vi "CPP-Multiplot.vi"(0 "PlotArray":cluster{dbl[], dbl[]}[](array[cluster]), 1 "Job Directory":path) -> (2 "Saved Automatically?":bool, 3 "gnuplotScript":string, 4 "Plot data file":path)   [LabVIEW 2015]
uses:
  gnuplotScriptComponents/plotstyle.ctl
  gnuplotScriptComponents/graphPeripherals.ctl
  gnuplotScriptComponents/minAndMax.ctl
  gnuplotScriptComponents/AutoManualNumber.ctl
  gnuplotScriptComponents/ticsAndGrids.ctl
  gnuplotScriptComponents/tics.ctl
  gnuplotScriptComponents/grids.ctl
  gnuplotScriptComponents/legendProperties.ctl
  gnuplotScriptComponents/legendAppearance.ctl
  gnuplotScriptComponents/alignment.ctl
  gnuplotScriptComponents/at.ctl
  gnuplotScriptComponents/margins.ctl
  gnuplotScriptComponents/source.ctl
  gnuplotScriptComponents/Master_Legend.ctl
  gnuplotScriptComponents/MasterPeripherals.ctl
  gnuplotScriptComponents/axisName.ctl
  Results_plotter_Global.vi
panel:
  in  "ThetaLabelCMD":string="rmax = GPVAL_R_MAX\nrmin = GPVAL_R_MIN\nThetaLabelPosn = rmax + (rmax - rmin) * 0.1\ndo for [jip = 0:17]{\nthetaer = jip*20\ntexter = sprintf(\"%.0f\",thetaer)\nset_label(x,text) = sprintf(\"set label '%s%s' at (-ThetaLabelPosn*cos(90+%f)), (ThetaLabelPosn*sin(90+%f)) center\", texter,\"$^{o}$\", thetaer, thetaer)\neval set_label(thetaer,texter)\n}\nset multiplot previous\n\nreplot\n\nunset label\n"
  out "Multi_Plot":bool
  in  "OpenLogfile?":bool
  in  "Show Script Editor?":bool
  in  "Tab Control":T1(tab)=enum."Appearance"
  in  "Each Graph contains:":T2=enum."Series"
  in  "Rows from:":T2=enum."Until done"
  in  "Columns from:":T2=enum."Selector 1"
  in  "Margins":T3={"Top"=2.0, "Bottom"=2.0, "Left"=2.0, "Right"=2.0}
  in  "Height (in)":dbl=7.0 min=0.5 step=0.5 format="%.1f"
  in  "Width (in)":dbl=10.0 min=0.5 step=0.5 format="%.1f"
  in  "nRows":u8=3 min=1
  in  "nCols":u8=3 min=1
  in  "ScaleAdjust":dbl=0.9 min=0.1 max=2.0 step=0.1
  in  "PlotTitlesNeed $$?":bool=TRUE
  in  "Show Channels with range of Values?":bool
  in  "ManualPlotTitles":string[](array[string])
  out "AutoPlotTitles":string[](array[string])
  in  "Individual Plot Titles":bool=TRUE
  in  "Page Title Pre Block":string
  in  "Page Title Post Block":string
  in  "Values to include in Page Title":i32[](listbox)
  in  "Plot Title Offset (characters)":cluster{"horizontal":dbl, "vertical":dbl}
  out "Final Title":string
  in  "PlotNamesNeed $$?":bool=TRUE
  in  "Plot Legends Manual":string[](array[string])
  in  "Plotstyles":T4[](array[typedef])=[{"Style"="linespoints", "Color"=16711680, "PointType"=1, "PointSize"=1.0, "LineWidth"=1.0, "LineType"=1}, {"Style"="linespoints", "Color"=16860, "PointType"=2, "PointSize"=1.0, "LineWidth"=1.0, "LineType"=1}, {"Style"="linespoints", "Color"=51228, "PointType"=3, "PointSize"=1.0, "LineWidth"=1.0, "LineType"=1}, {"Style"="linespoints", "Color"=0, "PointType"=4, "PointSize"=1.0, "LineWidth"=1.0, "LineType"=1}, {"Style"="linespoints", "Color"=9567230, "PointType"=5, "PointSize"=1.0, "LineWidth"=1.0, "LineType"=1}, {"Style"="linespoints", "Color"=12369084, "PointType"=6, "PointSize"=1.0, "LineWidth"=1.0, "LineType"=1}, {"Style"="linespoints", "Color"=15667967, "PointType"=7, "PointSize"=1.0, "LineWidth"=1.0, "LineType"=1}, {"Style"="linespoints", "Color"=15400704, "PointType"=8, "PointSize"=1.0, "LineWidth"=1.0, "LineType"=1}, {"Style"="linespoints", "Color"=128, "PointType"=9, "PointSize"=1.0, "LineWidth"=1.0, "LineType"=1}, {"Style"="linespoints", "Color"=8404992, "PointType"=10, "PointSize"=1.0, "LineWidth"=1.0, "LineType"=1}, {"Style"="linespoints", "Color"=6737151, "PointType"=11, "PointSize"=1.0, "LineWidth"=1.0, "LineType"=1}, {"Style"="linespoints", "Color"=8388672, "PointType"=12, "PointSize"=1.0, "LineWidth"=1.0, "LineType"=1}, {"Style"="linespoints", "Color"=16740303, "PointType"=13, "PointSize"=1.0, "LineWidth"=1.0, "LineType"=1}, {"Style"="linespoints", "Color"=16764006, "PointType"=14, "PointSize"=1.0, "LineWidth"=1.0, "LineType"=1}, {"Style"="linespoints", "Color"=8421376, "PointType"=15, "PointSize"=1.0, "LineWidth"=1.0, "LineType"=1}, {"Style"="linespoints", "Color"=65408, "PointType"=16, "PointSize"=1.0, "LineWidth"=1.0, "LineType"=1}] caption="Style                      Colour    PointType       PointSize         Linewidth        Linestyle" {"LineType" min=1 max=6 step=1; "LineWidth" min=1 max=6 step=1; "PointSize" min=0 step=0.1}
  out "Plot Legends Auto":string[](array[string])
  out "No of Series supplied":i32
  out "No of Graph Slots Available":i32
  in  "Plot Legends":bool=TRUE
  in  "X axis label":enum32{"Autolabel", "Manual Label"}(tab)
  out "X or theta label":string
  in  "X or theta label Manual":string
  in  "LegendProperties":T5={"Appearance"={"layout"="", "text-sample order"="", "key order"="", "surroundingBox"="", "MaxRows"=0, "MaxCols"=0, "WidthAdjust"=0.0}, "Alignment"={"Horizontal"="", "Vertical"=""}, "Location"="auto", "\"At\" location"={"XcoordSys"="", "YcoordSys"="", "Xvalue"=0.0, "Yvalue"=0.0}}
  in  "Y/R tics And Grids":T9={"tics"={"ticMin"=0.0, "ticStep"=5.0, "ticMax"=0.0, "minorDivsPerMajor"=2, "ticSpacing"=enum."Approx n Tics (rounded)", "ticPosition"=enum."Inside, no mirror"}, "Grids"={"Gridlines"=enum."No grids", "Zeroaxis"=enum."No zero axis"}, "Mapping"=enum."Lin"}
  in  "X/Theta tics And Grids":T9={"tics"={"ticMin"=0.0, "ticStep"=5.0, "ticMax"=0.0, "minorDivsPerMajor"=2, "ticSpacing"=enum."Approx n Tics (rounded)", "ticPosition"=enum."Inside, no mirror"}, "Grids"={"Gridlines"=enum."Major grid", "Zeroaxis"=enum."No zero axis"}, "Mapping"=enum."Lin"}
  in  "PlotType":enum32{"XY", "Polar", "Time"}(tab)
  in  "yAxisBounds":T12={"Min"={"Auto"=TRUE, "Value"=0.0}, "Max"={"Auto"=TRUE, "Value"=0.0}}
  in  "Additional XYgnuplot":string
  in  "xAxisBounds":T12={"Min"={"Auto"=TRUE, "Value"=0.0}, "Max"={"Auto"=TRUE, "Value"=0.0}}
  in  "Set bounds using XY Plot \non Results file plotter":bool
  in  "Angle Units":bool=TRUE
  in  "AngleMode":string(combo)="Compass"
  in  "wrapGapsUpTo:":dbl=30.0 step=0.1
  in  "Additional Polar gnuplot":string
  in  "rAxisBounds":T12={"Min"={"Auto"=FALSE, "Value"=0.0}, "Max"={"Auto"=FALSE, "Value"=1.5}}
  out "Time format?":bool
  in  "Time/Date Format":string(combo)="%I:%M %p\\n%d-%b-%y"
  in  "Select Time Zone":u32(ring)=142 items=["Abbreviation (Time Zone Name)", "A (Alpha Time Zone)", "ACDT (Australian Central Daylight Time  CDT – Central Daylight Time CDST – Central Daylight Savings Time)", "ACST (Australian Central Standard Time  CST – Central Standard Time)", "ACT (Acre Time)", "ACT (Australian Central Time)", "ACWST (Australian Central Western Standard Time)", "ADT (Arabia Daylight Time  AST – Arabia Summer Time)", "ADT (Atlantic Daylight Time  ADST – Atlantic Daylight Saving Time AST – Atlantic Summer Time  HAA – Heure Avancée de l'Atlantique (French))", "AEDT (Australian Eastern Daylight Time  EDT – Eastern Daylight Time EDST – Eastern Daylight Saving Time)", "AEST (Australian Eastern Standard Time  EST – Eastern Standard Time AET – Australian Eastern Time)", "AET (Australian Eastern Time)", "AFT (Afghanistan Time)", "AKDT (Alaska Daylight Time  ADST – Alaska Daylight Saving Time)", "AKST (Alaska Standard Time  AT – Alaska Time)", "ALMT (Alma-Ata Time)", "AMST (Amazon Summer Time)", "AMST (Armenia Summer Time  AMDT – Armenia Daylight Time)", "AMT (Amazon Time)", "AMT (Armenia Time)", "ANAST (Anadyr Summer Time)", "ANAT (Anadyr Time)", "AQTT (Aqtobe Time)", "ART (Argentina Time)", "AST (Arabia Standard Time  AST – Arabic Standard Time AST – Al Manamah Standard Time)", "AST (Atlantic Standard Time  AT – Atlantic Time  AST – Tiempo Estándar del Atlántico (Spanish) HNA – Heure Normale de l'Atlantique (French))", "AT (Atlantic Time)", "AWDT (Australian Western Daylight Time  WDT – Western Daylight Time WST – Western Summer Time)", "AWST (Australian Western Standard Time  WST – Western Standard Time WAT – Western Australia Time)", "AZOST (Azores Summer Time  AZODT – Azores Daylight Time)", "AZOT (Azores Time  AZOST – Azores Standard Time)", "AZST (Azerbaijan Summer Time)", "AZT (Azerbaijan Time)", "AoE (Anywhere on Earth)", "B (Bravo Time Zone)", "BNT (Brunei Darussalam Time  BDT – Brunei Time)", "BOT (Bolivia Time)", "BRST (Brasília Summer Time  BST – Brazil Summer Time BST – Brazilian Summer Time)", "BRT (Brasília Time  BT – Brazil Time BT – Brazilian Time)", "BST (Bangladesh Standard Time)", "BST (Bougainville Standard Time)", "BST (British Summer Time  BDT – British Daylight Time BDST – British Daylight Saving Time)", "BTT (Bhutan Time)", "C (Charlie Time Zone)", "CAST (Casey Time)", "CAT (Central Africa Time)", "CCT (Cocos Islands Time)", "CDT (Central Daylight Time  CDST – Central Daylight Saving Time NACDT – North American Central Daylight Time  HAC – Heure Avancée du Centre (French))", "CDT (Cuba Daylight Time)", "CEST (Central European Summer Time  CEDT – Central European Daylight Time ECST – European Central Summer Time  MESZ – Mitteleuropäische Sommerzeit (German))", "CET (Central European Time  ECT – European Central Time CET – Central Europe Time  MEZ – Mitteleuropäische Zeit (German))", "CHADT (Chatham Island Daylight Time  CDT – Chatham Daylight Time)", "CHAST (Chatham Island Standard Time)", "CHOST (Choibalsan Summer Time  CHODT – Choibalsan Daylight Time CHODST – Choibalsan Daylight Saving Time)", "CHOST (Choibalsan Summer Time)", "CHOT (Choibalsan Time)", "CHUT (Chuuk Time)", "CIDST (Cayman Islands Daylight Saving Time)", "CIST (Cayman Islands Standard Time  CIT – Cayman Islands Time)", "CKT (Cook Island Time)", "CLST (Chile Summer Time  CLDT – Chile Daylight Time)", "CLT (Chile Standard Time  CT – Chile Time CLST – Chile Standard Time)", "COT (Colombia Time)", "CST (Central Standard Time  CT – Central Time NACST – North American Central Standard Time  CST – Tiempo Central Estándar (Spanish) HNC – Heure Normale du Centre (French))", "CST (China Standard Time)", "CST (Cuba Standard Time)", "CT (Central Time)", "CVT (Cape Verde Time)", "CXT (Christmas Island Time)", "ChST (Chamorro Standard Time  GST – Guam Standard Time)", "D (Delta Time Zone)", "DAVT (Davis Time)", "DDUT (Dumont-d'Urville Time)", "E (Echo Time Zone)", "EASST (Easter Island Summer Time  EADT – Easter Island Daylight Time)", "EAST (Easter Island Standard Time)", "EAT (Eastern Africa Time  EAT – East Africa Time)", "ECT (Ecuador Time)", "EDT (Eastern Daylight Time  EDST – Eastern Daylight Savings Time NAEDT – North American Eastern Daylight Time  HAE – Heure Avancée de l'Est (French) EDT – Tiempo de verano del Este (Spanish))", "EEST (Eastern European Summer Time  EEDT – Eastern European Daylight Time  OESZ – Osteuropäische Sommerzeit (German))", "EET (Eastern European Time  OEZ – Osteuropäische Zeit (German))", "EGST (Eastern Greenland Summer Time  EGST – East Greenland Summer Time)", "EGT (East Greenland Time  EGT – Eastern Greenland Time)", "EST (Eastern Standard Time  ET – Eastern Time  NAEST – North American Eastern Standard Time  ET – Tiempo del Este (Spanish) HNE – Heure Normale de l'Est (French))", "ET (Eastern Time)", "F (Foxtrot Time Zone)", "FET (Further-Eastern European Time)", "FJST (Fiji Summer Time  FJDT – Fiji Daylight Time)", "FJT (Fiji Time)", "FKST (Falkland Islands Summer Time  FKDT – Falkland Island Daylight Time)", "FKT (Falkland Island Time  FKST – Falkland Island Standard Time)", "FNT (Fernando de Noronha Time)", "G (Golf Time Zone)", "GALT (Galapagos Time)", "GAMT (Gambier Time  GAMT – Gambier Islands Time)", "GET (Georgia Standard Time)", "GFT (French Guiana Time)", "GILT (Gilbert Island Time)", "GMT (Greenwich Mean Time  \"– Coordinated Universal Time GT – Greenwich Time)", "GST (Gulf Standard Time)", "GST (South Georgia Time)", "GYT (Guyana Time)", "H (Hotel Time Zone)", "HADT (Hawaii-Aleutian Daylight Time  HDT – Hawaii Daylight Time)", "HAST (Hawaii-Aleutian Standard Time  HST – Hawaii Standard Time)", "HKT (Hong Kong Time)", "HOVST (Hovd Summer Time  HOVDT – Hovd Daylight Time HOVDST – Hovd Daylight Saving Time)", "HOVST (Hovd Summer Time)", "HOVT (Hovd Time)", "I (India Time Zone)", "ICT (Indochina Time)", "IDT (Israel Daylight Time)", "IOT (Indian Chagos Time)", "IRDT (Iran Daylight Time  IRST – Iran Summer Time IDT – Iran Daylight Time)", "IRKST (Irkutsk Summer Time)", "IRKT (Irkutsk Time)", "IRST (Iran Standard Time  IT – Iran Time)", "IST (India Standard Time  IT – India Time IST – Indian Standard Time)", "IST (Irish Standard Time  IST – Irish Summer Time)", "IST (Israel Standard Time)", "JST (Japan Standard Time)", "K (Kilo Time Zone)", "KGT (Kyrgyzstan Time)", "KOST (Kosrae Time)", "KRAST (Krasnoyarsk Summer Time)", "KRAT (Krasnoyarsk Time)", "KST (Korea Standard Time  KST – Korean Standard Time KT – Korea Time)", "KUYT (Kuybyshev Time  SAMST – Samara Summer Time)", "L (Lima Time Zone)", "LHDT (Lord Howe Daylight Time)", "LHST (Lord Howe Standard Time)", "LINT (Line Islands Time)", "M (Mike Time Zone)", "MAGST (Magadan Summer Time  MAGST – Magadan Island Summer Time)", "MAGT (Magadan Time  MAGT – Magadan Island Time)", "MART (Marquesas Time)", "MAWT (Mawson Time)", "MDT (Mountain Daylight Time  MDST – Mountain Daylight Saving Time NAMDT – North American Mountain Daylight Time  HAR – Heure Avancée des Rocheuses (French))", "MHT (Marshall Islands Time)", "MMT (Myanmar Time)", "MSD (Moscow Daylight Time  Moscow Summer Time)", "MSK (Moscow Standard Time  MCK – Moscow Time)", "MST (Mountain Standard Time  MT – Mountain Time NAMST – North American Mountain Standard Time  HNR – Heure Normale des Rocheuses (French))", "MT (Mountain Time)", "MUT (Mauritius Time)", "MVT (Maldives Time)", "MYT (Malaysia Time  MST – Malaysian Standard Time)", "N (November Time Zone)", "NCT (New Caledonia Time)", "NDT (Newfoundland Daylight Time  HAT – Heure Avancée de Terre-Neuve (French))", "NFT (Norfolk Time  NFT – Norfolk Island Time)", "NOVST (Novosibirsk Summer Time  OMSST – Omsk Summer Time)", "NOVT (Novosibirsk Time  OMST – Omsk Standard Time)", "NPT (Nepal Time)", "NRT (Nauru Time)", "NST (Newfoundland Standard Time  HNT – Heure Normale de Terre-Neuve (French))", "NUT (Niue Time)", "NZDT (New Zealand Daylight Time)", "NZST (New Zealand Standard Time)", "O (Oscar Time Zone)", "OMSST (Omsk Summer Time  NOVST – Novosibirsk Summer Time)", "OMST (Omsk Standard Time  OMST – Omsk Time NOVT – Novosibirsk Time)", "ORAT (Oral Time)", "P (Papa Time Zone)", "PDT (Pacific Daylight Time  PDST – Pacific Daylight Saving Time NAPDT – North American Pacific Daylight Time  HAP – Heure Avancée du Pacifique (French))", "PET (Peru Time)", "PETST (Kamchatka Summer Time)", "PETT (Kamchatka Time  PETT – Petropavlovsk-Kamchatski Time)", "PGT (Papua New Guinea Time)", "PHOT (Phoenix Island Time)", "PHT (Philippine Time  PST – Philippine Standard Time)", "PKT (Pakistan Standard Time  PKT – Pakistan Time)", "PMDT (Pierre & Miquelon Daylight Time)", "PMST (Pierre & Miquelon Standard Time)", "PONT (Pohnpei Standard Time)", "PST (Pacific Standard Time  PT – Pacific Time NAPST – North American Pacific Standard Time  PT – Tiempo del Pacífico (Spanish) HNP – Heure Normale du Pacifique (French))", "PST (Pitcairn Standard Time)", "PT (Pacific Time)", "PWT (Palau Time)", "PYST (Paraguay Summer Time)", "PYT (Paraguay Time)", "PYT (Pyongyang Time  PYST – Pyongyang Standard Time)", "PYT (Pyongyang Time)", "Q (Quebec Time Zone)", "QYZT (Qyzylorda Time)", "R (Romeo Time Zone)", "RET (Reunion Time)", "ROTT (Rothera Time)", "S (Sierra Time Zone)", "SAKT (Sakhalin Time)", "SAMT (Samara Time  SAMT – Samara Standard Time)", "SAST (South Africa Standard Time  SAST – South African Standard Time)", "SBT (Solomon Islands Time  SBT – Solomon Island Time)", "SCT (Seychelles Time)", "SGT (Singapore Time  SST – Singapore Standard Time)", "SRET (Srednekolymsk Time)", "SRT (Suriname Time)", "SST (Samoa Standard Time)", "SYOT (Syowa Time)", "T (Tango Time Zone)", "TAHT (Tahiti Time)", "TFT (French Southern and Antarctic Time  KIT – Kerguelen (Islands) Time)", "TJT (Tajikistan Time)", "TKT (Tokelau Time)", "TLT (East Timor Time)", "TMT (Turkmenistan Time)", "TOT (Tonga Time)", "TVT (Tuvalu Time)", "U (Uniform Time Zone)", "ULAST (Ulaanbaatar Summer Time  ULAST – Ulan Bator Summer Time)", "ULAST (Ulaanbaatar Summer Time)", "ULAT (Ulaanbaatar Time  ULAT – Ulan Bator Time)", "ULAT (Ulaanbaatar Time)", "UTC (Coordinated Universal Time)", "UYST (Uruguay Summer Time)", "UYT (Uruguay Time)", "UZT (Uzbekistan Time)", "V (Victor Time Zone)", "VET (Venezuelan Standard Time  HLV – Hora Legal de Venezuela (Spanish))", "VLAST (Vladivostok Summer Time)", "VLAT (Vladivostok Time)", "VOST (Vostok Time)", "VUT (Vanuatu Time  EFATE – Efate Time)", "W (Whiskey Time Zone)", "WAKT (Wake Time)", "WARST (Western Argentine Summer Time)", "WAST (West Africa Summer Time)", "WAT (West Africa Time)", "WEST (Western European Summer Time  WEDT – Western European Daylight Time  WESZ – Westeuropäische Sommerzeit (German))", "WET (Western European Time  GMT – Greenwich Mean Time  WEZ – Westeuropäische Zeit (German))", "WFT (Wallis and Futuna Time)", "WGST (Western Greenland Summer Time  WGST – West Greenland Summer Time)", "WGT (West Greenland Time  WGT – Western Greenland Time)", "WIB (Western Indonesian Time  WIB – Waktu Indonesia Barat)", "WIT (Eastern Indonesian Time  WIT – Waktu Indonesia Timur)", "WITA (Central Indonesian Time  WITA – Waktu Indonesia Tengah)", "WST (West Samoa Time  ST – Samoa Time)", "WST (Western Sahara Summer Time)", "WT (Western Sahara Standard Time  WT – Western Sahara Time)", "X (X-ray Time Zone)", "Y (Yankee Time Zone)", "YAKST (Yakutsk Summer Time)", "YAKT (Yakutsk Time)", "YAPT (Yap Time)", "YEKST (Yekaterinburg Summer Time)", "YEKT (Yekaterinburg Time)", "Z (Zulu Time Zone)"]
  out "Time Format String":string="%I:%M %p\\n%d-%b-%y"
  out "Formatted date/time string":string="05:00 PM\\n21-Jan-16"
  out "TZ Shift (hrs)":string="UTC-7.00"
  in  "Y axis label":enum32{"Autolabel", "Manual Label"}(tab)
  out "Y or R label":string
  in  "Y or R label Manual 2":string
  in  "PeripheralsMasterControl":T14=enum."Edges Only"
  in  "Legend Options":T15=enum."Single Legend Below table"
  in  "GraphPeripherals":T16[][](array[typedef])
  out "PlotCommand":string
  in  "Filename Max length":i32=255
  out "File Path Control":path
  out "AuditTrail":string[](array[string])
  out "Desired Legends":string[][](array[string])
  out "original name had conflict":bool
  out "crossplatform problem":bool
  # "Rows/ Columns/ Series from: controls not wired- just a thought for explicit control of what goes where...?"
  # "Overall Page Title"
  # "There are as many graphs as there are titles (from Selector 2)...."
  # "Plot Styles"
  # "Each graph contains plots from Selector 1..."
  # "X/theta"
  # "Y/r"
  # "Shows the numbered line colours and point styles available- well it would, if it didn't disappear every time I update from the repository..!"
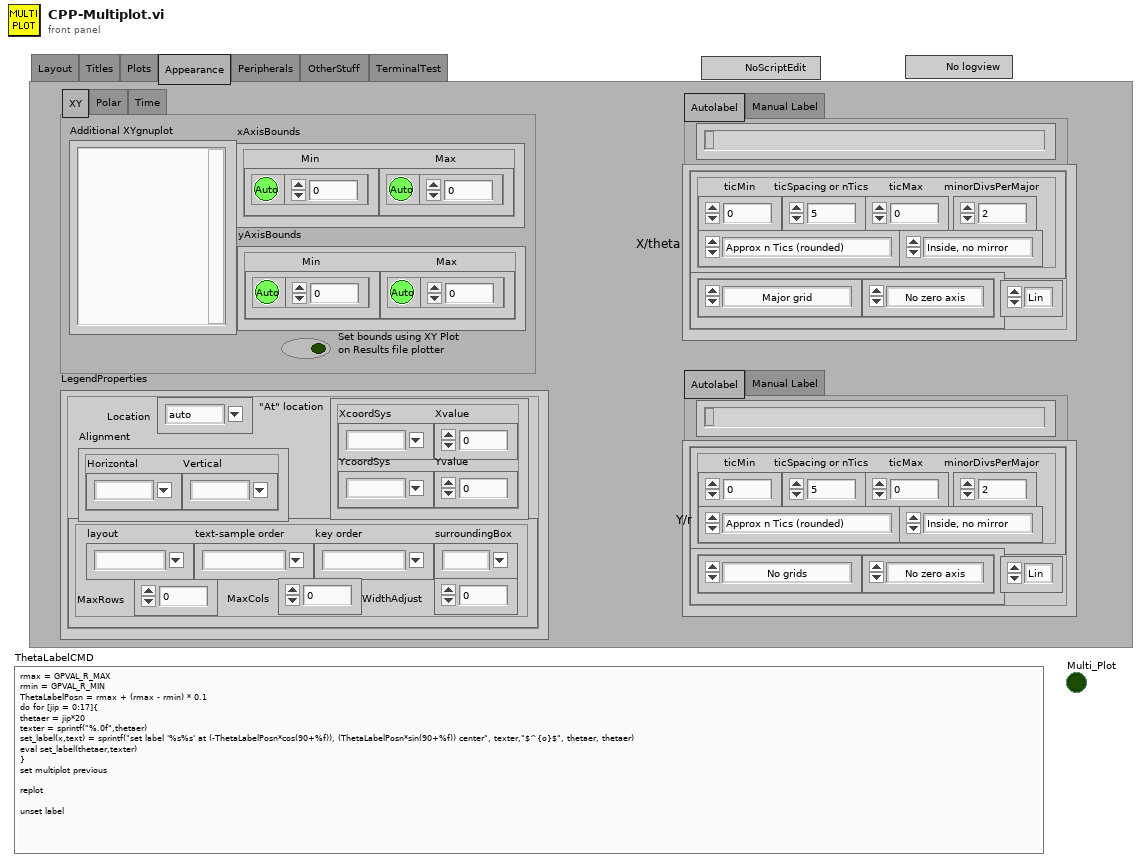
[diagram p1: front panel]
types:
  T1 = enum32{"Layout", "Titles", "Plots", "Appearance", "Peripherals", "OtherStuff ", "TerminalTest"}
  T2 = typedef "source.ctl" = enum16{"Specified:", "Selector 1", "Selector 2", "Until done", "Series"}
  T3 = typedef "margins.ctl" = cluster{"Top":dbl, "Bottom":dbl, "Left":dbl, "Right":dbl}
  T4 = typedef "plotstyle.ctl" = cluster{"Style":string, "Color":u32, "PointType":i32, "PointSize":sgl, "LineWidth":sgl, "LineType":u8}
  T5 = typedef "legendProperties.ctl" = cluster{"Appearance":T6, "Alignment":T7, "Location":string, "\"At\" location":T8}
  T6 = typedef "legendAppearance.ctl" = cluster{"layout":string, "text-sample order":string, "key order":string, "surroundingBox":string, "MaxRows":u32, "MaxCols":u32, "WidthAdjust":dbl}
  T7 = typedef "alignment.ctl" = cluster{"Horizontal":string, "Vertical":string}
  T8 = typedef "at.ctl" = cluster{"XcoordSys":string, "YcoordSys":string, "Xvalue":dbl, "Yvalue":dbl}
  T9 = typedef "ticsAndGrids.ctl" = cluster{"tics":T10, "Grids":T11, "Mapping":enum8{"Lin", "Log"}}
  T10 = typedef "tics.ctl" = cluster{"ticMin":dbl, "ticStep":dbl, "ticMax":dbl, "minorDivsPerMajor":i32, "ticSpacing":enum16{"Auto Tics", "Fixed spacing", "Fixed Minimum and Spacing", "Start, Spacing and Maximum", "Approx n Tics (rounded)"}, "ticPosition":enum16{"Inside, no mirror", "Inside, mirrored", "Outside, no mirror", "Outside, mirrored", "Invisible"}}
  T11 = typedef "grids.ctl" = cluster{"Gridlines":enum16{"No grids", "Major grid", "Minor grid", "Major and Minor"}, "Zeroaxis":enum16{"No zero axis", "Show zero axis"}}
  T12 = typedef "minAndMax.ctl" = cluster{"Min":T13, "Max":T13}
  T13 = typedef "AutoManualNumber.ctl" = cluster{"Auto":bool, "Value":dbl}
  T14 = typedef "MasterPeripherals.ctl" = enum16{"Use Table", "Titles On", "Edges Only", "All Off"}
  T15 = typedef "Master_Legend.ctl" = enum16{"No Legend", "Single Legend Below table", "Legend as per array"}
  T16 = typedef "graphPeripherals.ctl" = cluster{"title":bool, "key":bool, "Xtic":bool, "Ytic":bool, "Xlab":bool, "Ylab":bool}
  T17 = typedef "axisName.ctl" = string
  T18 = typedef "LVDateTimeRec.ctl" = cluster{"fractional second":dbl, "second":i32, "minute":i32, "hour":i32, "day of month":i32, "month":i32, "year":i32, "day of week":i32, "day of year":i32, "DST":i32}
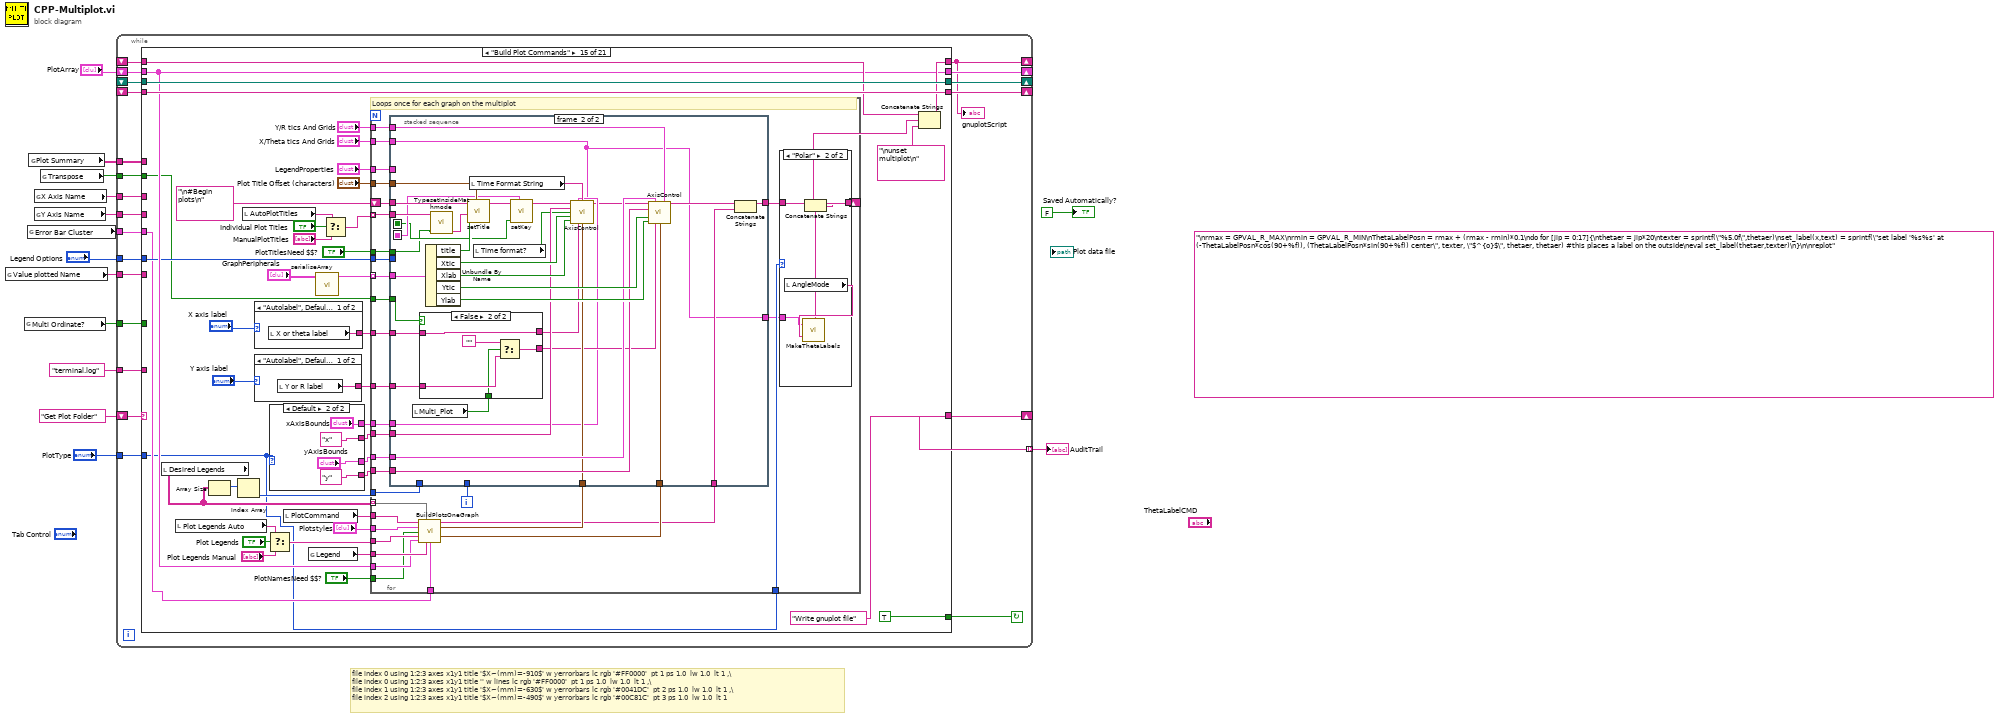
[diagram p0: block diagram]
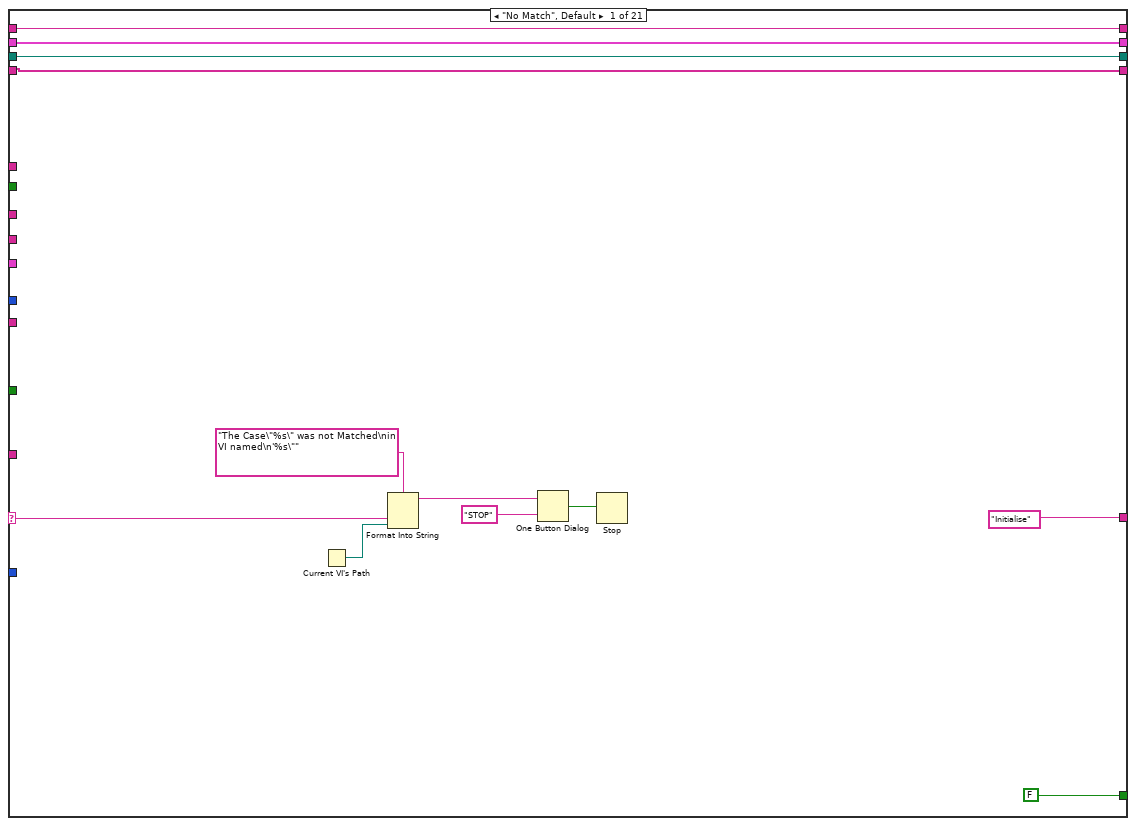
[diagram p2: hidden frame]
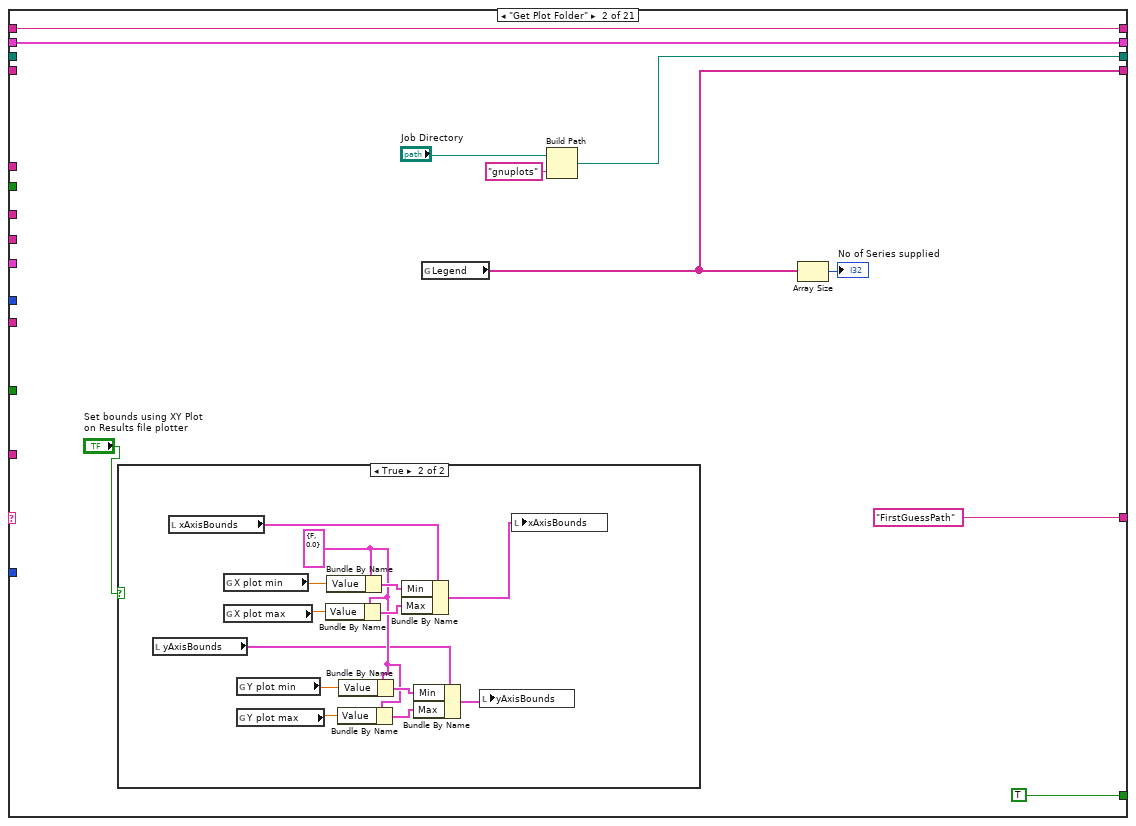
[diagram p3: hidden frame]
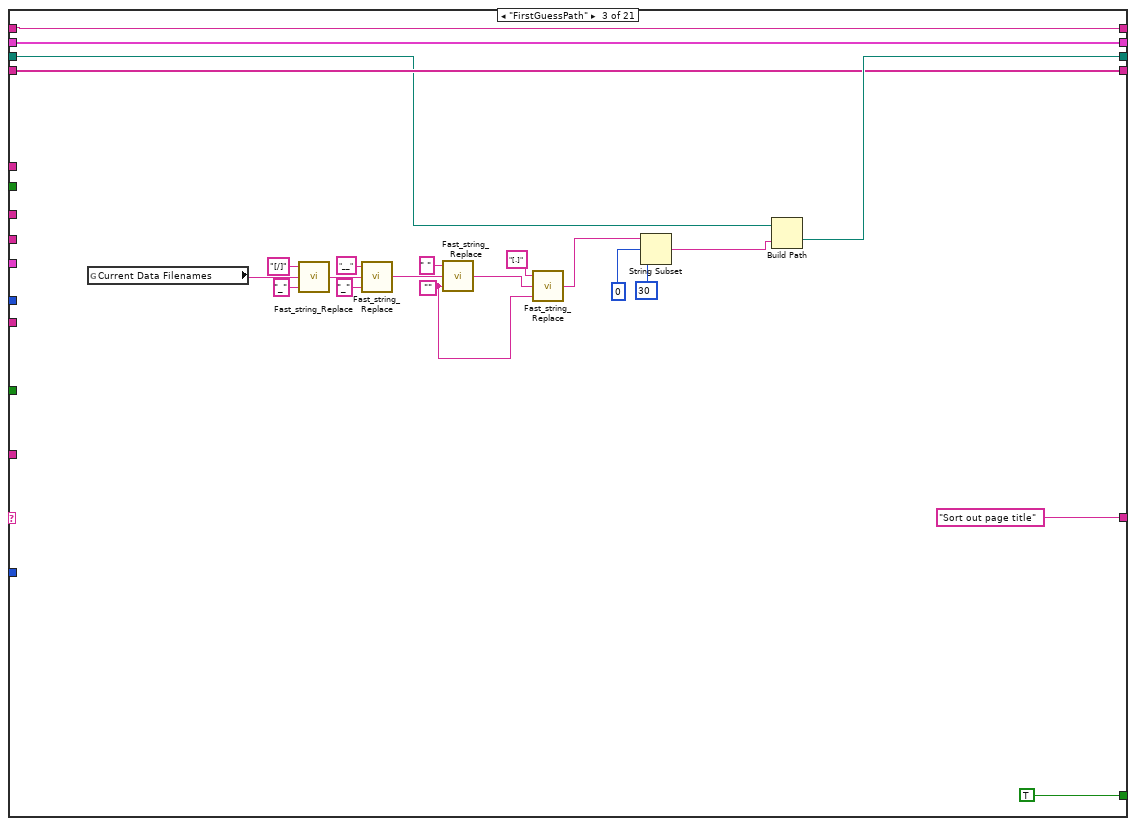
[diagram p5: hidden frame]
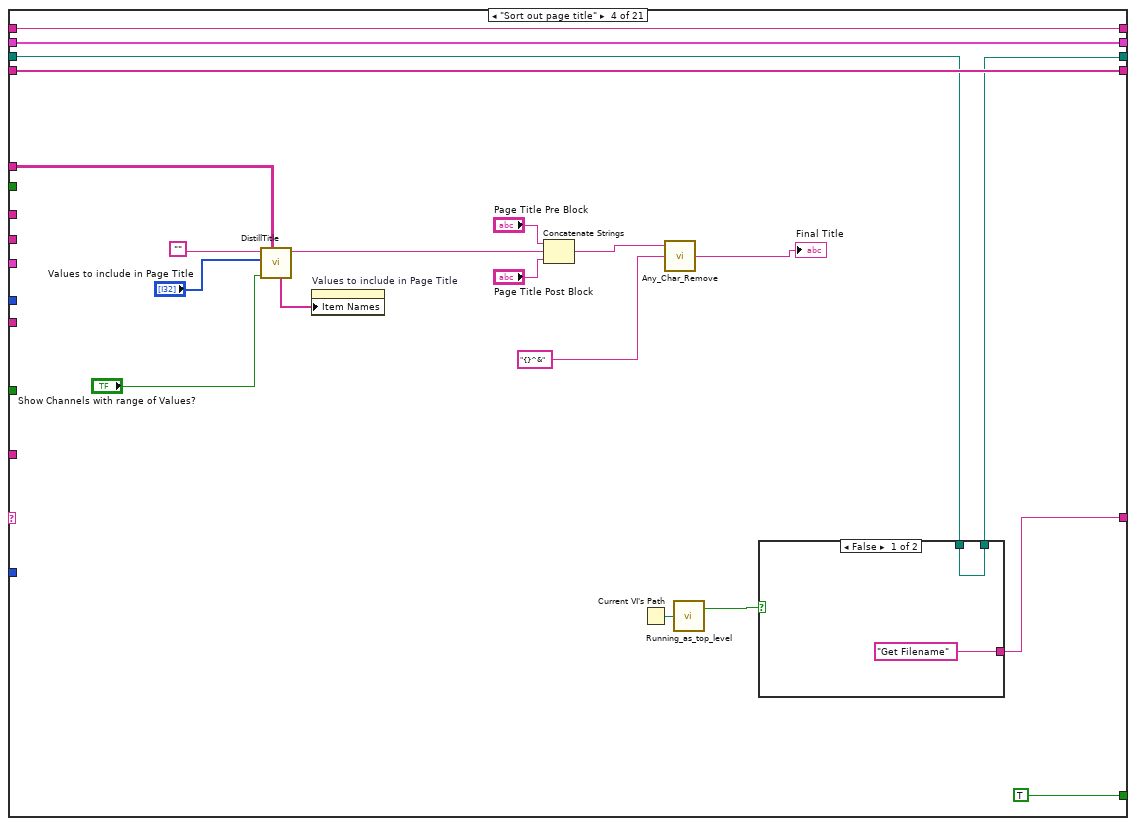
[diagram p6: hidden frame]
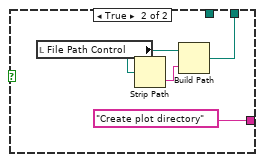
[diagram p7: hidden frame]
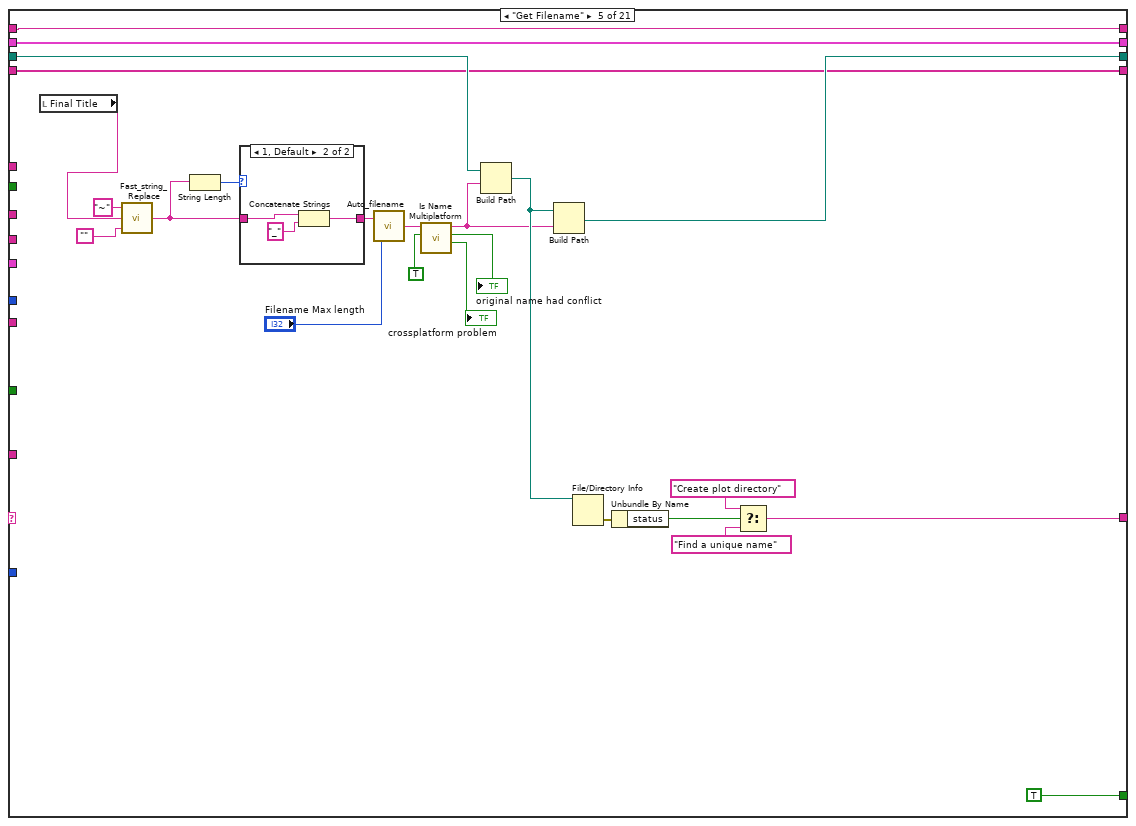
[diagram p8: hidden frame]
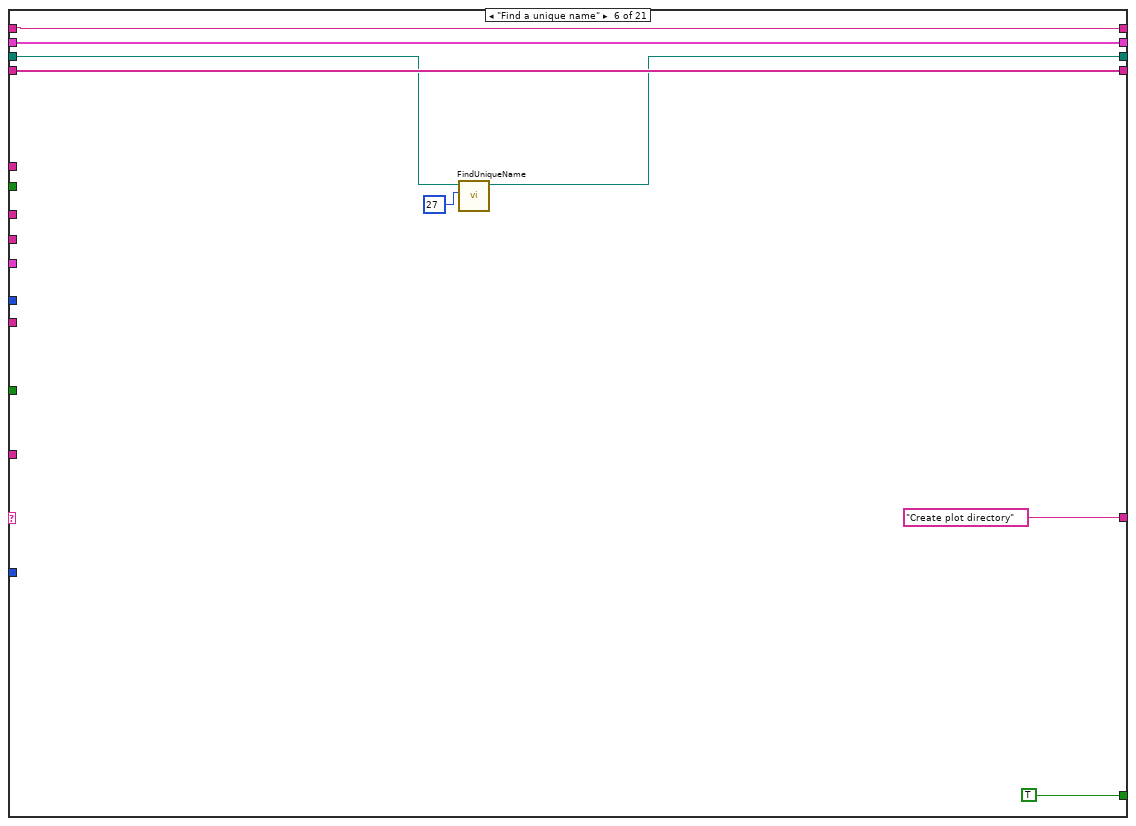
[diagram p10: hidden frame]
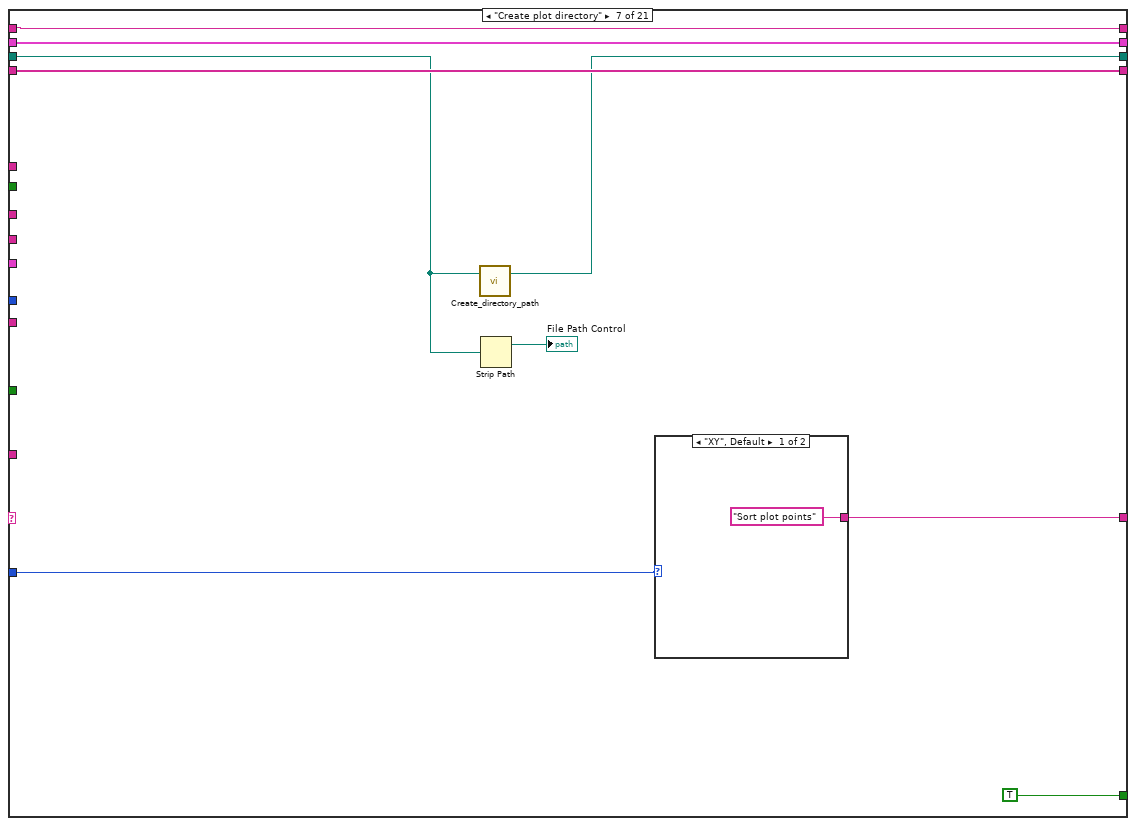
[diagram p11: hidden frame]
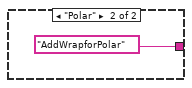
[diagram p12: hidden frame]
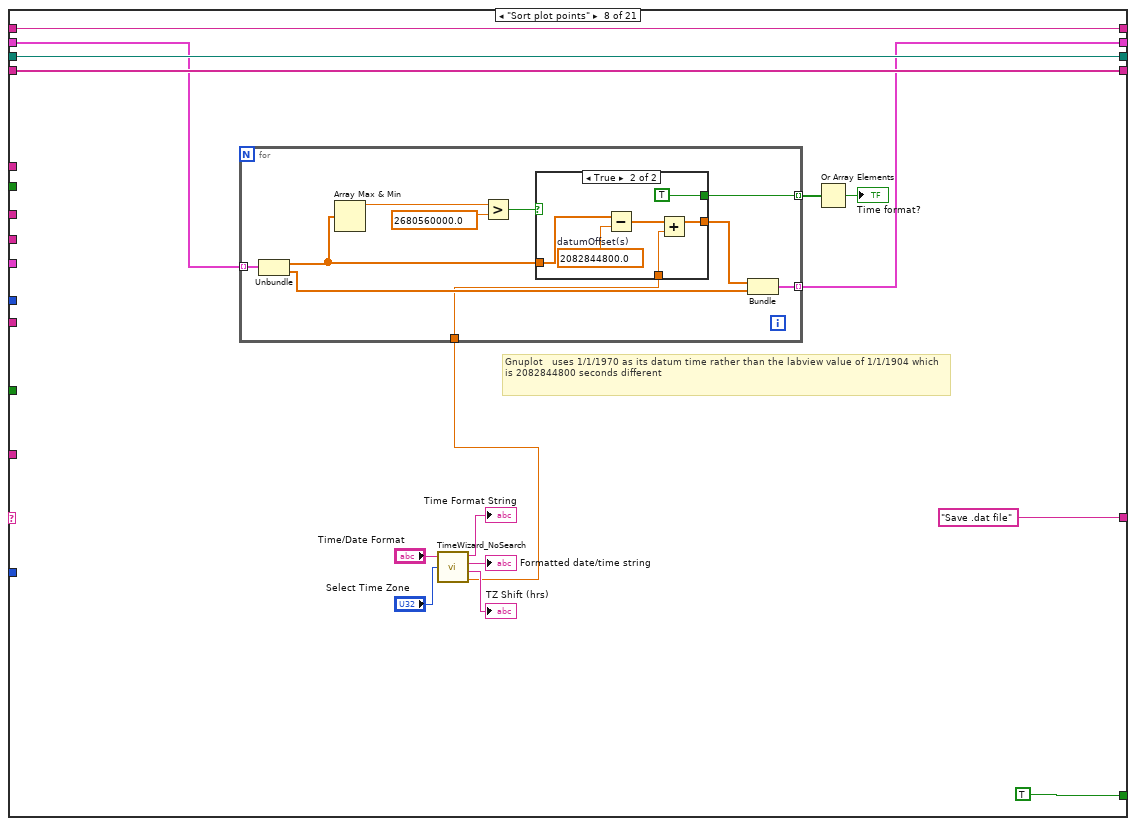
[diagram p13: hidden frame]
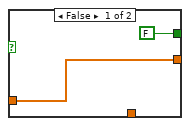
[diagram p14: hidden frame]
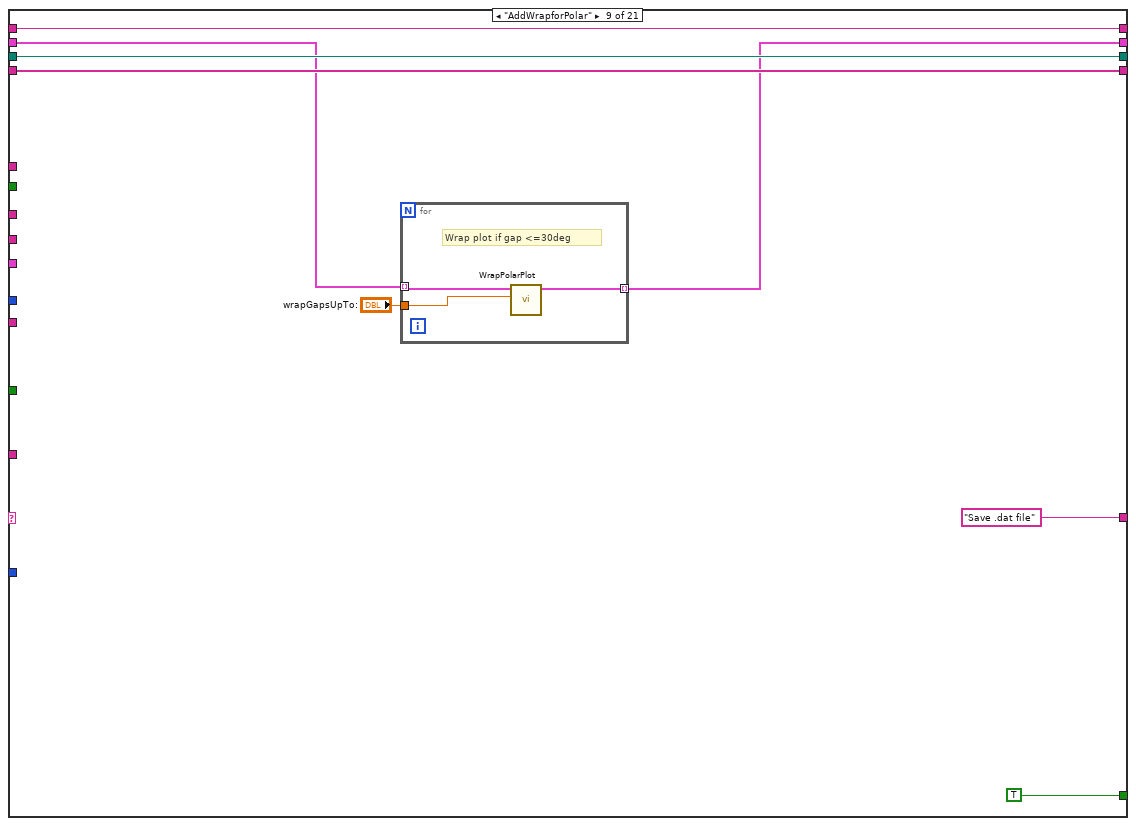
[diagram p15: hidden frame]
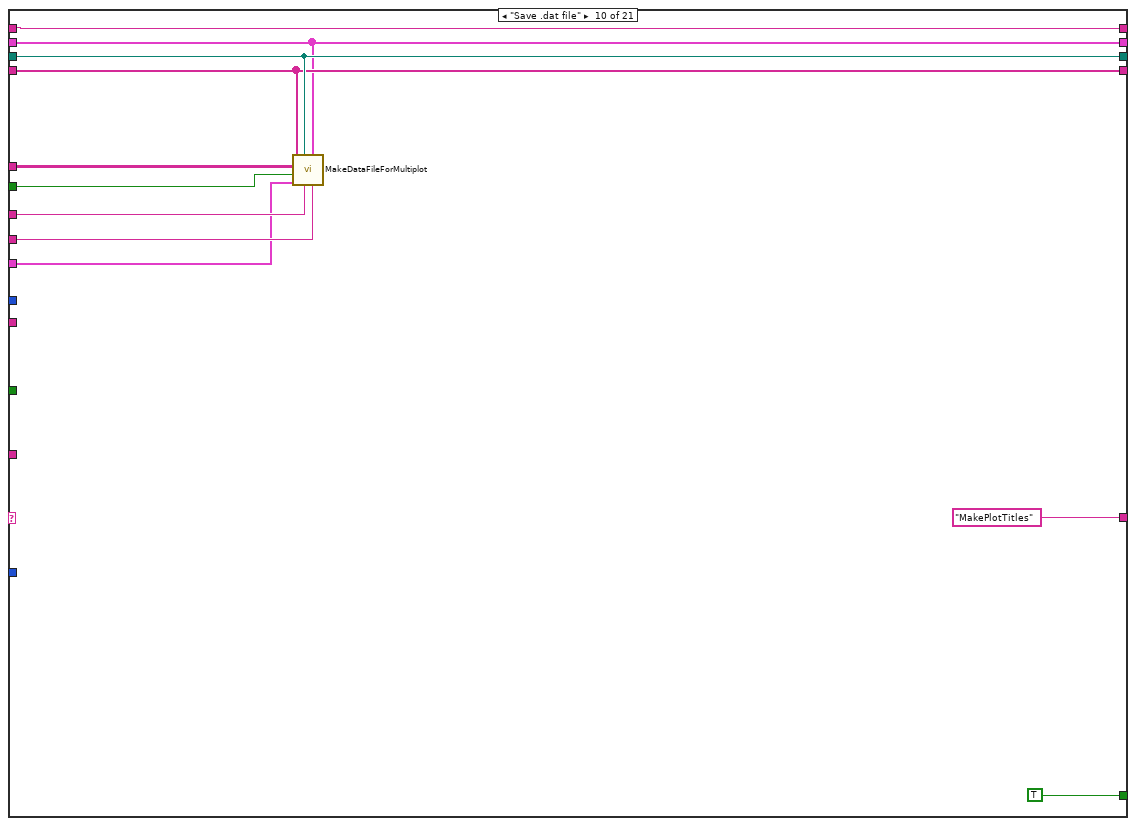
[diagram p16: hidden frame]
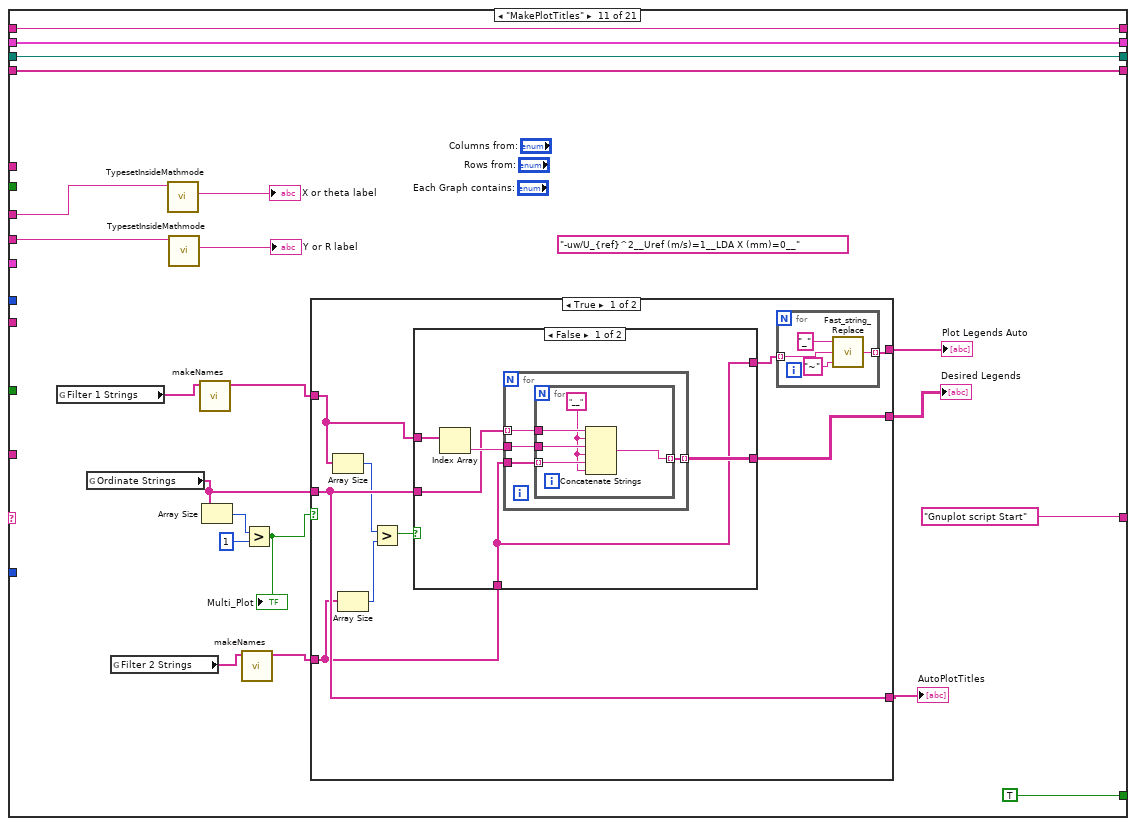
[diagram p17: hidden frame]
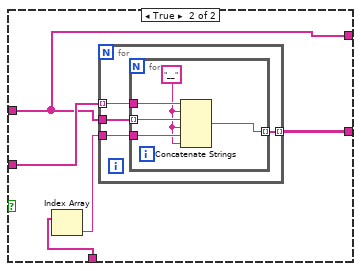
[diagram p18: hidden frame]
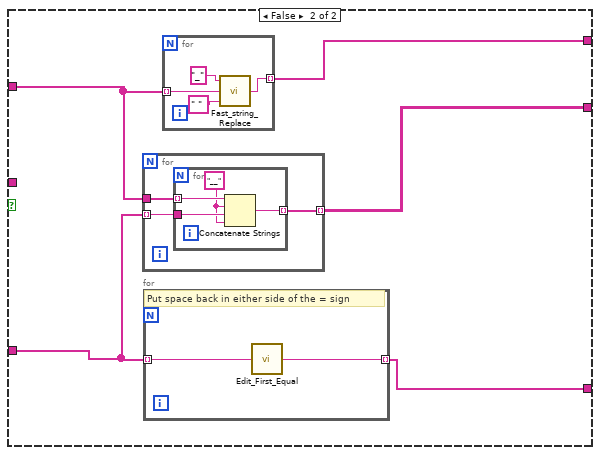
[diagram p19: hidden frame]
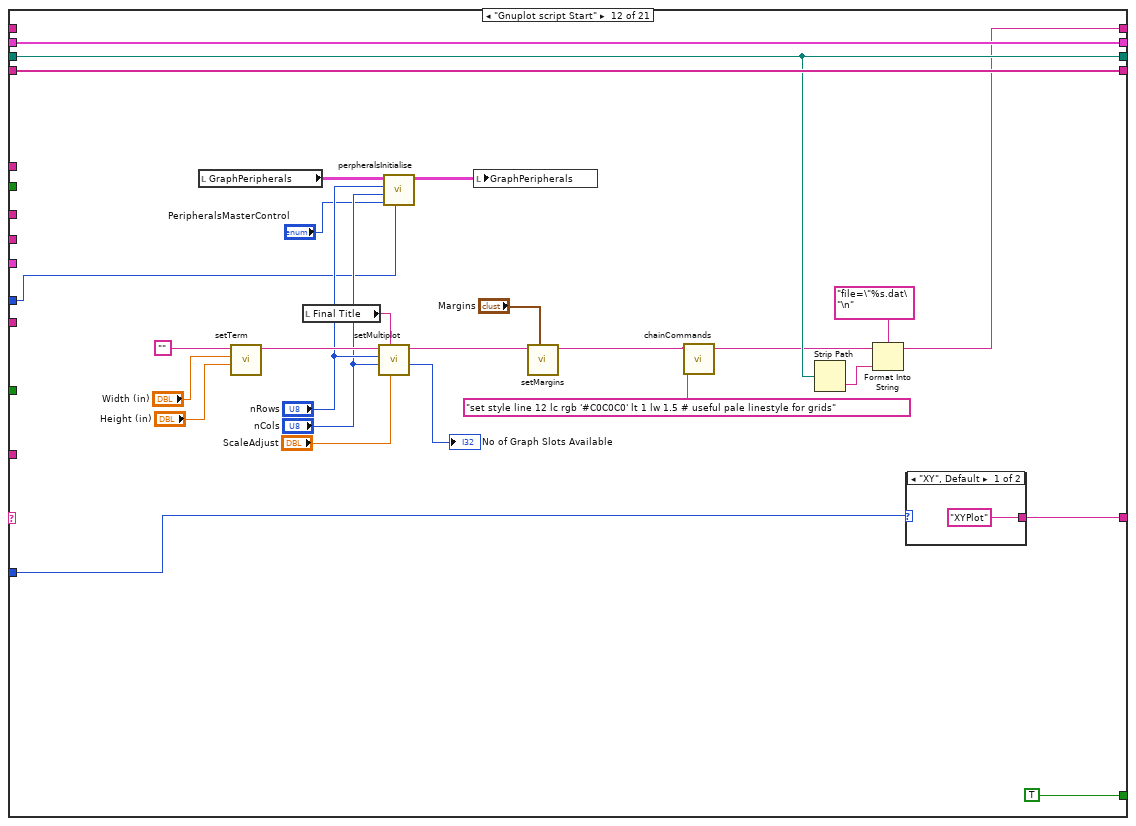
[diagram p20: hidden frame]
diagram:
  (unwired) "\nrmax = GPVAL_R_MAX\nrmin = GPVAL_R_MIN\nThetaLabelPosn = rmax + (rmax - rmin)*0.1\ndo for [jip = 0:17]{\nthetaer = jip*20\ntexter = sprintf(\"%5.0f\",thetaer)\nset_label(x,text) = sprintf(\"set label '%s%s' at (-ThetaLabelPosn*cos(90+%f)), (ThetaLabelPosn*sin(90+%f)) center\", texter, \"$^{o}$\", thetaer, thetaer) #this places a label on the outside\neval set_label(thetaer,texter)\n}\n\nreplot" ("string")
  # "file index 0 using 1:2:3 axes x1y1 title '$X~(mm)=-910$' w yerrorbars lc rgb '#FF0000'  pt 1 ps 1.0  lw 1.0  lt 1 ,\\\nfile index 0 using 1:2:3 axes x1y1 title '' w lines lc rgb '#FF0000'  pt 1 ps 1.0  lw 1.0  lt 1 ,\\\nfile index 1 using 1:2:3 axes x1y1 title '$X~(mm)=-630$' w yerrorbars lc rgb '#0041DC'  pt 2 ps 1.0  lw 1.0  lt 1 ,\\\nfile index 2 using 1:2:3 axes x1y1 title '$X~(mm)=-490$' w yerrorbars lc rgb '#00C81C'  pt 3 ps 1.0  lw 1.0  lt 1"
  n1 = global read "Results_plotter_Global.vi" "Value plotted Name"() -> (w10:string)
  n2 = global read "Results_plotter_Global.vi" "Multi Ordinate?"() -> (w6:bool)
  n3 = global read "Results_plotter_Global.vi" "Error Bar Cluster"() -> (w1:cluster{string[]}[])
  n4 = global read "Results_plotter_Global.vi" "Plot Summary"() -> (w13:string[][])
  n5 = global read "Results_plotter_Global.vi" "X Axis Name"() -> (w12:string)
  n6 = global read "Results_plotter_Global.vi" "Y Axis Name"() -> (w11:string)
  n7 = global read "Results_plotter_Global.vi" "Transpose"() -> (w7:bool)
  n8 = while {
    shift-left: "Get Plot Folder" -> [w34]
    shift-right: [w18] -> _
    tunnel: w13 -> [w33]
    shift-right: [w32] -> _
    shift-left: _ -> [w31]
    tunnel: w12 -> [w30]
    tunnel: w11 -> [w29]
    tunnel: w10 -> [w28]
    shift-right: [w26] -> _
    shift-left: "PlotArray" -> [w27]
    shift-right: [w19] -> _
    shift-left: _ -> [w25]
    shift-right: [w24] -> _
    shift-left: _ -> [w23]
    tunnel: "terminal.log" -> [w22]
    tunnel: w7 -> [w21]
    tunnel: w6 -> [w20]
    tunnel: [w18] -> w5 mode=indexing
    tunnel: "PlotType" -> [w17]
    tunnel: "Legend Options" -> [w16]
    tunnel: w1 -> [w15]
    stop <- w35 continue-if-true
    n9 = case shown="\"Build Plot Commands\"" w34 {
      selector: w34 -> [w36 _ _ _ _ _ _ _ _ _ _ _ _ _ _ _ _ _ _ _ _]
      tunnel: [FALSE TRUE TRUE ("Top Level") TRUE ("Top Level") TRUE ("Top Level") TRUE ("Top Level") TRUE TRUE TRUE ("Top Level") TRUE ("Top Level") TRUE ("Top Level") TRUE ("Top Level") TRUE ("Top Level") TRUE ("Top Level") TRUE ("Top Level") TRUE ("Top Level") TRUE ("Top Level") TRUE ("Top Level") FALSE ("Top Level") TRUE ("Top Level") FALSE ("Top Level")] -> w35
      tunnel: ["Initialise" "FirstGuessPath" "Sort out page title" w104 w140 "Create plot directory" w155 "Save .dat file" "Save .dat file" "MakePlotTitles" "Gnuplot script Start" w324 "Build Plot Commands" "Build Plot Commands" "Write gnuplot file" ("t") "Execute shell script" ("t") "Has pdf been generated?" ("t") w602 "End" "End" ("t") "End" ("t")] -> w18
      tunnel: w33 -> [_ _ _ w99 _ _ _ _ _ w218 _ _ _ _ _ _ _ _ _ _ _]
      tunnel: [w40 w55 w92 w106 w141 w147 w160 w180 w205 w219 w241 w315 w340 w366 w420 w560 w568 w597 w615 w625 w636] -> w32
      tunnel: w31 -> [w40 _ w88 w105 w137 w148 w159 w180 w205 w219 w241 w315 w340 w366 w420 w560 w568 w597 w615 w625 w636]
      tunnel: w30 -> [_ _ _ _ _ _ _ _ _ w217 w235 _ _ _ _ _ _ _ _ _ _]
      tunnel: w29 -> [_ _ _ _ _ _ _ _ _ w216 w234 _ _ _ _ _ _ _ _ _ _]
      tunnel: w28 -> [_ _ _ _ _ _ _ _ _ _ _ _ _ _ _ _ _ _ _ _ _]
      tunnel: w27 -> [w39 w51 w91 w112 w139 w151 w163 w175 w201 w213 w240 w327 w339 w367 w388 w566 w573 w608 w620 w630 w635]
      tunnel: [w39 w51 w91 w112 w139 w151 w163 w174 w200 w213 w240 w327 w339 w367 w388 w566 w573 w608 w620 w630 w635] -> w26
      tunnel: w25 -> [w38 w54 w90 w110 w138 w150 w162 w179 w206 w220 w239 _ w333 w361 w412 w556 w571 w606 w618 w628 w634]
      tunnel: [w38 w54 w90 w110 w138 w150 w162 w179 w206 w220 w239 w301 w335 w362 w418 w556 w571 w606 w618 w628 w634] -> w19
      tunnel: [w37 w50 w89 w111 w136 w149 w161 w178 w204 w215 w238 w326 w338 w365 w419 w561 w572 w607 w619 w629 w633] -> w24
      tunnel: w23 -> [w37 _ w89 w111 w136 w149 w161 w178 w204 w215 w238 w326 w338 w365 w419 w561 w572 w607 w619 w629 w633]
      tunnel: w22 -> [_ _ _ _ _ _ _ _ _ _ _ _ _ _ _ _ w567 _ _ w623 _]
      tunnel: w21 -> [_ _ _ _ _ _ _ _ _ w214 _ _ _ _ w384 _ _ _ _ _ _]
      tunnel: w20 -> [_ _ _ _ _ _ _ _ _ _ _ _ _ _ _ _ _ _ _ _ _]
      tunnel: w17 -> [_ _ _ _ _ _ w156 _ _ _ _ w302 _ _ w377 _ _ _ _ _ _]
      tunnel: w16 -> [_ _ _ _ _ _ _ _ _ _ _ w304 _ _ w387 _ _ _ _ _ _]
      tunnel: w15 -> [_ _ _ _ _ _ _ _ _ w210 _ _ _ _ w385 _ _ _ _ _ _]
      frame "No Match", Default {
        n10 = Current VI's Path() -> (path=w42:path)
        n11 = Format Into String(format string="The Case\"%s\" was not Matched\nin VI named\n'%s\"" ("Format String"), w36, w42) -> (resulting string=w45:string)  [unwired: 2 in, 1 out]
        n12 = One Button Dialog(message=w45, button name ("OK")="STOP") -> (true=w43:bool)
        n13 = Stop(stop? (T)=w43) -> ()
      }
      frame "Get Plot Folder" {
        n14 = case shown="True" "Set bounds using XY Plot \non Results file plotter" {
          frame False {
          }
          frame True {
            w60 = T13 {"Auto"=FALSE, "Value"=0.0} ("Min")
            n15 = local read "yAxisBounds"() -> (w59:T12)
            n16 = local read "xAxisBounds"() -> (w70:T12)
            n17 = global read "Results_plotter_Global.vi" "X plot min"() -> (w65:dbl)
            n18 = global read "Results_plotter_Global.vi" "X plot max"() -> (w66:dbl)
            n19 = global read "Results_plotter_Global.vi" "Y plot min"() -> (w64:dbl)
            n20 = global read "Results_plotter_Global.vi" "Y plot max"() -> (w63:dbl)
            n21 = Bundle By Name(cluster=w60, "Value"=w66) -> (w68:T13)
            n22 = Bundle By Name(cluster=w60, "Value"=w65) -> (w69:T13)
            n23 = Bundle By Name(cluster=w60, "Value"=w63) -> (w62:T13)
            n24 = Bundle By Name(cluster=w60, "Value"=w64) -> (w61:T13)
            n25 = Bundle By Name(cluster=w70, "Min"=w69, "Max"=w68) -> (w67:T12)
            n26 = Bundle By Name(cluster=w59, "Min"=w61, "Max"=w62) -> (w58:T12)
            n27 = local write "yAxisBounds"(w58) -> ()
            n28 = local write "xAxisBounds"(w67) -> ()
          }
        }
        n29 = global read "Results_plotter_Global.vi" "Legend"() -> (w50:string[])
        n30 = Build Path(base path="Job Directory", name or relative path="gnuplots") -> (appended path=w55:path)
        n31 = Array Size(array=w50) -> (size(s)=→"No of Series supplied":i32)
      }
      frame "FirstGuessPath" {
        w74 = ""
        n32 = global read "Results_plotter_Global.vi" "Current Data Filenames"() -> (w78:string)
        n33 = call "Fast_string_Replace.vi"("Replace match with:"="_", "Input String"=w78, "regular expression"="[/]") -> ("Output String"=w81:string)  [unwired: 2 out]
        n34 = call "Fast_string_Replace.vi"("Replace match with:"="_", "Input String"=w81, "regular expression"="__") -> ("Output String"=w79:string)  [unwired: 2 out]
        n35 = call "Fast_string_Replace.vi"("Replace match with:"=w74, "Input String"=w79, "regular expression"=" ") -> ("Output String"=w73:string)  [unwired: 2 out]
        n36 = call "Fast_string_Replace.vi"("Replace match with:"=w74, "Input String"=w73, "regular expression"="[.]") -> ("Output String"=w72:string)  [unwired: 2 out]
        n37 = String Subset(string=w72, offset (0)=0, length (rest)=30 ("length (rest)")) -> (substring=w71:string)
        n38 = Build Path(base path=w88, name or relative path=w71) -> (appended path=w92:path)
      }
      frame "Sort out page title" {
        n39 = call "DistillTitle.vi"("Plot Summary in"=w99, "Show Channels with range of Values?"="Show Channels with range of Values?", "Indices to include in Page Title"="Values to include in Page Title", "String in"="") -> ("String out"=w103:string, "AvailableVariables"=w97:string[])  [unwired: 6 in]
        n40 = property on="Values to include in Page Title" class="LstBox (strict)"("Item Names"=w97) -> ()  [unwired: 2 in, 2 out]
        n41 = Concatenate Strings("Page Title Pre Block", w103, "Page Title Post Block") -> (w96:string)
        n42 = Current VI's Path() -> (path=w109:path)
        n43 = call "Any_Char_Remove.vi"("Individual Characters to Remove"="{}^&", "String in"=w96) -> ("String out"=→"Final Title":string)  [unwired: 1 in]
        n44 = call "Running_as_top_level.vi"("Vi path name"=w109) -> ("Top Level"=w107:bool)  [unwired: 1 out]
        n45 = case shown="False" w107 {
          tunnel: [w114 w117] -> w106
          tunnel: w105 -> [w114 _]
          tunnel: ["Get Filename" ("t") "Create plot directory"] -> w104
          frame False {
          }
          frame True {
            n46 = local read "File Path Control"() -> (w116:path)
            n47 = Strip Path(path=w116) -> (name=w115:string)  [unwired: 1 out]
            n48 = Build Path(base path=w116, name or relative path=w115) -> (appended path=w117:path)
          }
        }
      }
      frame "Get Filename" {
        n49 = local read "Final Title"() -> (w126:string)
        n50 = call "Fast_string_Replace.vi"("Replace match with:"="", "Input String"=w126, "regular expression"="~") -> ("Output String"=w123:string)  [unwired: 1 in, 1 out]
        n51 = String Length(string=w123) -> (length=w128:i32)
        n52 = case shown="1, Default" w128 {
          tunnel: [w143 w144] -> w127
          tunnel: w123 -> [w143 w146]
          frame 0 {
          }
          frame 1, Default {
            n53 = Concatenate Strings(w146, "_") -> (w144:string)
          }
        }
        n54 = call "Auto_filename.vi"("Filename Max length"="Filename Max length", "Prefix"=w127) -> ("Filename"=w130:string)
        n55 = call <vilib>:"Is Name Multiplatform.vi"("name must work for all platforms (F)"=TRUE, "filename"=w130) -> ("crossplatform problem"=→"crossplatform problem":bool, "original name had conflict"=→"original name had conflict":bool, "suggested filename"=w122:string)  [unwired: 5 in, 2 out]
        n56 = Build Path(base path=w137, name or relative path=w122) -> (appended path=w134:path)
        n57 = Build Path(base path=w134, name or relative path=w122) -> (appended path=w141:path)
        n58 = File/Directory Info(path=w134) -> (error out=w135:errorcluster)  [unwired: 1 in, 6 out]
        n59 = Unbundle By Name(w135) -> ("status"=w133:bool)
        n60 = Select(t="Create plot directory", s=w133, f="Find a unique name") -> (s? t:f=w140:string)
      }
      frame "Find a unique name" {
        n61 = call "FindUniqueName.vi"("Max Length"=27, "PathIn"=w148) -> ("UniquedPath"=w147:path)  [unwired: 9 in]
      }
      frame "Create plot directory" {
        n62 = call "Create_directory_path.vi"("Path name"=w159) -> ("Path name Out"=w160:path)  [unwired: 1 in, 1 out]
        n63 = Strip Path(path=w159) -> (stripped path=→"File Path Control":path)  [unwired: 1 out]
        n64 = case shown="\"XY\", Default" w156 {
          tunnel: ["Sort plot points" "AddWrapforPolar"] -> w155
          frame "XY", Default {
          }
          frame "Polar" {
          }
        }
      }
      frame "Sort plot points" {
        # "Gnuplot   uses 1/1/1970 as its datum time rather than the labview value of 1/1/1904 which is 2082844800 seconds different"
        n65 = call "TimeWizard_NoSearch.vi"("Time/Date Format"="Time/Date Format", "Select Time Zone"="Select Time Zone") -> ("Format String"=→"Time Format String":string, "Formatted date/time string"=→"Formatted date/time string":string, "TZ Shift (hrs)"=→"TZ Shift (hrs)":string, "TZ Shift (sec)"=w166:dbl)  [unwired: 1 in]
        n66 = for {
          tunnel: w175 -> [w189] mode=indexing
          tunnel: [w190] -> w174 mode=indexing
          tunnel: [w182] -> w177 mode=indexing
          tunnel: w166 -> [w181]
          n67 = Unbundle(w189) -> ("Angle"=w185:dbl[], "Radius"=w186:dbl[])
          n68 = Array Max & Min(array=w185) -> (max value=w188:dbl)  [unwired: 3 out]
          n69 = Greater?(x=w188, y=2680560000.0) -> (0:w183:bool)
          n70 = case shown="True" w183 {
            tunnel: w185 -> [w192 w198]
            tunnel: [w192 w194] -> w184
            tunnel: [FALSE TRUE] -> w182
            tunnel: w181 -> [_ w193]
            frame False {
            }
            frame True {
              w197 = 2082844800.0  # datumOffset(s)
              n71 = Subtract(x=w198, y=w197) -> (x-y=w196:dbl[])
              n72 = Add(x=w196, y=w193) -> (x+y=w194:dbl[])
            }
          }
          n73 = Bundle("Angle"=w184, "Radius"=w186) -> (w190:cluster{"Angle":dbl[], "Radius":dbl[]})  [unwired: 1 out]
        }
        n74 = Or Array Elements(Boolean array=w177) -> (logical OR=→"Time format?":bool)
      }
      frame "AddWrapforPolar" {
        n75 = for {
          tunnel: w201 -> [w209] mode=indexing
          tunnel: [w208] -> w200 mode=indexing
          tunnel: "wrapGapsUpTo:" -> [w207]
          # "Wrap plot if gap <=30deg"
          n76 = call "WrapPolarPlot.vi"("maxWrap"=w207, "thetaRin"=w209) -> ("thetaRout"=w208:cluster{"Angle":dbl[], "Radius":dbl[]})  [unwired: 9 in]
        }
      }
      frame "Save .dat file" {
        n77 = call "MakeDataFileForMultiplot.vi"("Y Axis Name"=w216, "Plot Array"=w213, "X Axis Name"=w217, "Path"=w219, "Error Bar Cluster"=w210, "Transpose"=w214, "Plot Summary"=w218, "Legend"=w215) -> ()  [unwired: 4 in]
      }
      frame "MakePlotTitles" {
        (unwired) "-uw/U_{ref}^2__Uref (m/s)=1__LDA X (mm)=0__"
        n78 = global read "Results_plotter_Global.vi" "Filter 1 Strings"() -> (w221:string[])
        n79 = global read "Results_plotter_Global.vi" "Ordinate Strings"() -> (w228:string[])
        n80 = global read "Results_plotter_Global.vi" "Filter 2 Strings"() -> (w224:string[])
        n81 = call "TypesetInsideMathmode.vi"("DirtyString"=w235) -> ("Mathmode String"=→"X or theta label":string)  [unwired: 8 in, 2 out]
        n82 = call "TypesetInsideMathmode.vi"("DirtyString"=w234) -> ("Mathmode String"=→"Y or R label":string)  [unwired: 8 in, 2 out]
        n83 = call "makeNames.vi"("Strings"=w221) -> ("Names"=w222:string[])  [unwired: 10 in]
        n84 = Array Size(array=w228) -> (size(s)=w227:i32)
        n85 = call "makeNames.vi"("Strings"=w224) -> ("Names"=w223:string[])  [unwired: 10 in]
        n86 = Greater?(x=w227, y=1) -> (0:w225:bool)
        "Multi_Plot" <- w225
        n87 = case shown="True" w225 {
          tunnel: w222 -> [w245 w283]
          tunnel: w223 -> [w246 w284]
          tunnel: [w242 w287] -> w231
          tunnel: [w249 w286] -> w230
          tunnel: [w250 w285] -> w229
          tunnel: w228 -> [w249 _]
          frame True {
            n88 = Array Size(array=w245) -> (size(s)=w248:i32)
            n89 = Array Size(array=w246) -> (size(s)=w247:i32)
            n90 = Greater?(x=w248, y=w247) -> (0:w244:bool)
            n91 = case shown="False" w244 {
              tunnel: [w258 w273] -> w250
              tunnel: w249 -> [w257 w272]
              tunnel: w246 -> [w255 w271]
              tunnel: w245 -> [w256 w269]
              tunnel: [w255 w269] -> w243
              frame False {
                n92 = Index Array(array=w256) -> (element=w259:string)  [unwired: 1 in]
                n93 = for {
                  tunnel: w259 -> [w263]
                  tunnel: w255 -> [w262]
                  tunnel: [w261] -> w258 mode=indexing
                  tunnel: w257 -> [w260] mode=indexing
                  n94 = for {
                    tunnel: w263 -> [w268]
                    tunnel: w262 -> [w267] mode=indexing
                    tunnel: [w266] -> w261 mode=indexing
                    tunnel: w260 -> [w265]
                    w264 = "__" ("string")
                    n95 = Concatenate Strings(w265, w264, w268, w264, w267, w264) -> (w266:string)
                  }
                }
              }
              frame True {
                n96 = Index Array(array=w271) -> (element=w270:string)  [unwired: 1 in]
                n97 = for {
                  tunnel: w269 -> [w277]
                  tunnel: w270 -> [w276]
                  tunnel: [w275] -> w273 mode=indexing
                  tunnel: w272 -> [w274] mode=indexing
                  n98 = for {
                    tunnel: w277 -> [w282] mode=indexing
                    tunnel: w276 -> [w281]
                    tunnel: [w280] -> w275 mode=indexing
                    tunnel: w274 -> [w279]
                    w278 = "__" ("string")
                    n99 = Concatenate Strings(w279, w278, w282, w278, w281, w278) -> (w280:string)
                  }
                }
              }
            }
            n100 = for {
              tunnel: w243 -> [w253] mode=indexing
              tunnel: [w252] -> w242 mode=indexing
              n101 = call "Fast_string_Replace.vi"("Replace match with:"="~", "Input String"=w253, "regular expression"="_") -> ("Output String"=w252:string)  [unwired: 1 in, 1 out]
            }
          }
          frame False {
            n102 = for {
              tunnel: w283 -> [w296]
              tunnel: w284 -> [w295] mode=indexing
              tunnel: [w294] -> w285 mode=indexing
              n103 = for {
                tunnel: w296 -> [w300] mode=indexing
                tunnel: w295 -> [w299]
                tunnel: [w297] -> w294 mode=indexing
                w298 = "__" ("string")
                n104 = Concatenate Strings(w300, w298, w299, w298) -> (w297:string)
              }
            }
            n105 = for {
              tunnel: w284 -> [w293] mode=indexing
              tunnel: [w292] -> w286 mode=indexing
              # "Put space back in either side of the = sign"
              n106 = call "Edit_First_Equal.vi"("String in"=w293) -> ("String out"=w292:string)
            }
            n107 = for {
              tunnel: w283 -> [w289] mode=indexing
              tunnel: [w288] -> w287 mode=indexing
              n108 = call "Fast_string_Replace.vi"("Replace match with:"=" ", "Input String"=w289, "regular expression"="_") -> ("Output String"=w288:string)  [unwired: 2 out]
            }
          }
        }
        "AutoPlotTitles" <- w230
        "Plot Legends Auto" <- w231
        "Desired Legends" <- w229
      }
      frame "Gnuplot script Start" {
        n109 = local read "GraphPeripherals"() -> (w309:T16[][])
        n110 = call "setTerm.vi"("Height (in)"="Height (in)", "Width (in)"="Width (in)", "String in"="") -> ("String out"=w320:string)  [unwired: 7 in, 1 out]
        n111 = local read "Final Title"() -> (w318:string)
        n112 = call "setMultiplot.vi"("ScaleAdjust"="ScaleAdjust", "OverallTitle"=w318, "Cols"="nCols", "Rows"="nRows", "String in"=w320) -> ("nGraphs"=→"No of Graph Slots Available":i32, "String out"=w319:string)  [unwired: 4 in, 1 out]
        n113 = call "perpheralsInitialise.vi"("Legend"=w304, "PeripheralsMasterControl"="PeripheralsMasterControl", "Cols"="nCols", "Rows"="nRows", "GraphPeripheralsIn"=w309) -> ("GraphPeripheralsOut"=w310:T16[][])  [unwired: 6 in]
        n114 = local write "GraphPeripherals"(w310) -> ()
        n115 = call "setMargins.vi"("Margins"="Margins", "String in"=w319) -> ("String out"=w306:string)  [unwired: 8 in, 1 out]
        n116 = call "chainCommands.vi"("Command"="set style line 12 lc rgb '#C0C0C0' lt 1 lw 1.5 # useful pale linestyle for grids", "StringIn"=w306) -> ("StringOut"=w307:string)  [unwired: 9 in]
        n117 = Strip Path(path=w315) -> (name=w314:string)  [unwired: 1 out]
        n118 = Format Into String(format string="file=\"%s.dat\"\n" ("string"), initial string=w307, w314) -> (resulting string=w301:string)  [unwired: 1 in, 1 out]
        n119 = case shown="\"XY\", Default" w302 {
          tunnel: ["XYPlot" "PolarPlot"] -> w324
          frame "XY", Default {
          }
          frame "Polar" {
          }
        }
      }
      frame "XYPlot" {
        n120 = case shown="\"True\"" "Additional XYgnuplot" {
          selector: "Additional XYgnuplot" -> [w341 w345]
          tunnel: [w341 w344] -> w331
          frame "", Default {
          }
          frame "True" {
            n121 = Concatenate Strings("# Manual gnuplot Start" ("string"), w345, "# Manual gnuplot End" ("string")) -> (w344:string)
          }
        }
        n122 = Concatenate Strings(w333, "set border ls 12\n" ("input 2"), w331) -> (w335:string)
        "PlotCommand" <- "file index %d using 1:2 axes x1y1 title '%s' w " ("format string")
      }
      frame "PolarPlot" {
        n123 = case shown="\"True\"" "Additional Polar gnuplot" {
          selector: "Additional Polar gnuplot" -> [w370 w374]
          tunnel: [w370 w373] -> w350
          frame "", Default {
          }
          frame "True" {
            n124 = Concatenate Strings("# Manual gnuplot Start" ("string"), w374, "# Manual gnuplot End" ("string")) -> (w373:string)
          }
        }
        n125 = Select(t="set angles degrees\n", s="Angle Units", f="set angles radians\n") -> (s? t:f=w352:string)
        n126 = case shown="\"Compass\"" "AngleMode" {
          tunnel: ["90-$1" ("format string") "$1" ("format string")] -> w357
          frame "Compass" {
          }
          frame "Math", Default {
          }
        }
        n127 = Concatenate Strings(w361, w352, "set polar\nset size square\n", w350) -> (w362:string)
        n128 = case shown="\"Compass\"" "AngleMode" {
          tunnel: [90.0 0.0] -> w347
          frame "Compass" {
          }
          frame "Math", Default {
          }
        }
        n129 = Concatenate Strings("file index %d using (" ("format string"), w357, "):2 axes x1y1 title '%s' w " ("format string")) -> (w356:string)
        n130 = local read "X/Theta tics And Grids"() -> (w349:T9)
        n131 = Bundle By Name(cluster=w349, "tics.ticMin"=w347) -> (w348:T9)
        n132 = local write "PlotCommand"(w356) -> ()
        n133 = local write "X/Theta tics And Grids"(w348) -> ()
      }
      frame "Build Plot Commands" {
        n134 = local read "Desired Legends"() -> (w383:string[][])
        n135 = local read "Plot Legends Auto"() -> (w390:string[])
        n136 = Array Size(array=w383) -> (size(s)=w382:i32[])
        n137 = Index Array(array=w382) -> (element=w381:i32)  [unwired: 1 in]
        n138 = local read "AutoPlotTitles"() -> (w410:string[])
        n139 = case shown="\"Autolabel\", Default" "Y axis label" {
          tunnel: [w421 "Y or R label Manual 2"] -> w395
          frame "Autolabel", Default {
            n140 = local read "Y or R label"() -> (w421:string)
          }
          frame "Manual Label" {
          }
        }
        n141 = case shown="\"Autolabel\", Default" "X axis label" {
          tunnel: [w430 "X or theta label Manual"] -> w400
          frame "Autolabel", Default {
            n142 = local read "X or theta label"() -> (w430:string)
          }
          frame "Manual Label" {
          }
        }
        n143 = Select(t=w390, s="Plot Legends", f="Plot Legends Manual") -> (s? t:f=w389:string[])
        n144 = case shown="Default" w377 {
          tunnel: [T17 "theta" ("Axis") T17 "x" ("Axis")] -> w398
          tunnel: [T17 "r" ("Axis") T17 "y" ("Axis")] -> w397
          tunnel: ["rAxisBounds" "yAxisBounds"] -> w399
          tunnel: ["rAxisBounds" "xAxisBounds"] -> w378
          frame "Polar" {
          }
          frame Default {
          }
        }
        n145 = local read "PlotCommand"() -> (w402:string)
        n146 = global read "Results_plotter_Global.vi" "Legend"() -> (w406:string[])
        n147 = call "serialiseArray.vi"("GraphPeripherals"="GraphPeripherals") -> ("output array"=w407:T16[])  [unwired: 10 in]
        n148 = Select(t=w410, s="Individual Plot Titles", f="ManualPlotTitles") -> (s? t:f=w386:string[])
        n149 = for {
          shift-right: [w434] -> w413
          shift-left: "\n#Begin plots\n" -> [w462]
          tunnel: w389 -> [w463]
          tunnel: "Plotstyles" -> [w464]
          tunnel: w386 -> [w458] mode=indexing
          tunnel: w407 -> [w461] mode=indexing
          tunnel: w383 -> [w460] mode=indexing
          tunnel: w406 -> [w459]
          tunnel: "LegendProperties" -> [w447]
          tunnel: "Plot Title Offset (characters)" -> [w457]
          tunnel: w402 -> [w456]
          tunnel: w400 -> [w455]
          tunnel: w399 -> [w454]
          tunnel: w398 -> [w453]
          tunnel: w397 -> [w452]
          tunnel: w395 -> [w451]
          tunnel: "Y/R tics And Grids" -> [w450]
          tunnel: "X/Theta tics And Grids" -> [w449]
          tunnel: w388 -> [w448]
          tunnel: w387 -> [w446]
          tunnel: w385 -> [w442]
          tunnel: w384 -> [w441]
          tunnel: w381 -> [w440]
          tunnel: "PlotNamesNeed $$?" -> [w439]
          tunnel: "PlotTitlesNeed $$?" -> [w438]
          tunnel: w378 -> [w437]
          tunnel: w377 -> [w433]
          i -> [w445]
          # "Loops once for each graph on the multiplot"
          n150 = call "BuildPlotsOneGraph.vi"("PlotCommand"=w456, "Desired Legends"=w460, "Plotstyles"=w464, "PlotNamesNeed $$?"=w439, "Plot Legends"=w463, "PlotArray"=w448, "Legend"=w459, "Error Bar Cluster"=w442) -> ("String out"=w435:string, "Xspan"=w443:cluster{"Max":dbl, "Min":dbl}, "Yspan"=w444:cluster{"Max":dbl, "Min":dbl})  [unwired: 5 in]
          n151 = stacked-sequence {
            seq-local: [w477 _] -> [_ w530]
            seq-local: [w473 _] -> [_ w529]
            tunnel: [_ w545] -> w436
            tunnel: w435 -> [_ w544]
            tunnel: w462 -> [_ w543]
            tunnel: w461 -> [w475 w542]
            tunnel: w458 -> [_ w535]
            tunnel: w457 -> [_ w534]
            tunnel: w455 -> [_ w521]
            tunnel: w454 -> [_ w528]
            tunnel: w453 -> [_ w533]
            tunnel: w452 -> [_ w532]
            tunnel: w451 -> [_ w525]
            tunnel: w450 -> [_ w531]
            tunnel: w449 -> [_ w511]
            tunnel: w447 -> [w476 _]
            tunnel: w446 -> [w478 _]
            tunnel: w445 -> [w472 _]
            tunnel: w444 -> [_ w526]
            tunnel: w443 -> [_ w527]
            tunnel: w441 -> [_ w520]
            tunnel: w440 -> [w471 _]
            tunnel: w438 -> [_ w518]
            tunnel: w437 -> [_ w515]
            tunnel: [_ w511] -> w432
            frame #0 {
              n152 = Unbundle By Name(w475) -> ("key"=w474:bool)
              n153 = case shown="\"Single Legend Below table\"" w478 {
                tunnel: [w480 w484] -> w477
                tunnel: w476 -> [w480 w485]
                tunnel: w474 -> [w479 _]
                tunnel: [w479 w483] -> w473
                tunnel: w472 -> [_ w481]
                tunnel: w471 -> [_ w482]
                frame "Legend as per array", Default {
                }
                frame "Single Legend Below table" {
                  n154 = stacked-sequence {
                    seq-local: [w487 _] -> [_ w504]
                    seq-local: [w486 _] -> [_ w503]
                    tunnel: w485 -> [_ w510]
                    tunnel: w481 -> [_ w507]
                    tunnel: [_ w506] -> w484
                    tunnel: [_ w505] -> w483
                    tunnel: w482 -> [w489 _]
                    frame #0 {
                      n155 = local read "No of Graph Slots Available"() -> (w490:i32)
                      n156 = Greater?(x=w490, y=w489) -> (0:w488:bool)
                      n157 = case shown="False" w488 {
                        tunnel: [0.6 ("\"At\" location.Xvalue") w497] -> w487
                        tunnel: [-0.03 ("\"At\" location.Yvalue") w494] -> w486
                        frame False {
                        }
                        frame True {
                          n158 = local read "nCols"() -> (w501:u8)
                          n159 = local read "nRows"() -> (w495:u8)
                          n160 = Decrement(x=w501) -> (x-1=w502:u8)
                          n161 = Increment(x=w495) -> (x+1=w493:u8)
                          n162 = Divide(x=w502, y=w501) -> (x/y=w498:dbl)
                          n163 = Divide(x=1.0, y=w493) -> (x/y=w494:dbl)
                          n164 = Divide(x=0.7, y=w501) -> (x/y=w499:dbl)
                          n165 = Add(x=w498, y=w499) -> (x+y=w497:dbl)
                        }
                      }
                    }
                    frame #1 {
                      w508 = "screen" ("\"At\" location.XcoordSys")
                      # "Use \"screen\" coordinates to place legend at bottom-center\nof entire \"screen\" of graphs; update legend cluster to \nreflect this."
                      # "Only legend the first graph"
                      n166 = Equal To 0?(x=w507) -> (x = 0?=w505:bool)
                      n167 = Bundle By Name(cluster=w510, "Location"="at", "\"At\" location.XcoordSys"=w508, "\"At\" location.Xvalue"=w504, "\"At\" location.YcoordSys"=w508, "\"At\" location.Yvalue"=w503) -> (w506:T5)
                      n168 = local write "LegendProperties"(w506) -> ()
                    }
                  }
                }
              }
            }
            frame #1 {
              n169 = local read "Multi_Plot"() -> (w523:bool)
              n170 = case shown="False" w520 {
                tunnel: w525 -> [w546 w555]
                tunnel: [w546 w554] -> w524
                tunnel: w523 -> [w549 w552]
                tunnel: [w547 w551] -> w522
                tunnel: w521 -> [w548 w551]
                frame True {
                  n171 = Select(t="", s=w549, f=w548) -> (s? t:f=w547:string)
                }
                frame False {
                  n172 = Select(t="", s=w552, f=w555) -> (s? t:f=w554:string)
                }
              }
              n173 = Unbundle By Name(w542) -> ("title"=w541:bool, "Xtic"=w539:bool, "Xlab"=w538:bool, "Ytic"=w537:bool, "Ylab"=w536:bool)
              n174 = call "TypesetInsideMathmode.vi"("Needs $$?"=w518, "DirtyString"=w535) -> ("ChosenStringtype"=w519:string)  [unwired: 7 in, 2 out]
              n175 = call "setTitle.vi"("Offset"=w534, "Set?"=w541, "Title"=w519, "String in"=w543) -> ("String out"=w540:string)  [unwired: 6 in, 1 out]
              n176 = local read "Time Format String"() -> (w516:string)
              n177 = local read "Time format?"() -> (w517:bool)
              n178 = call "setKey.vi"("LegendProperties"=w530, "Set?"=w529, "String in"=w540) -> ("String out"=w514:string)  [unwired: 7 in, 1 out]
              n179 = call "AxisControl.vi"("String in"=w514, "AxisBounds"=w515, "Time Format String"=w516, "ticsAndGrids"=w511, "Axis"=w533, "Time format?"=w517, "ShowNumbers?"=w539, "ShowLabel?"=w538, "Axis Label"=w522, "DataSpan"=w527) -> ("String out"=w513:string)  [unwired: 4 in, 1 out]
              n180 = call "AxisControl.vi"("String in"=w513, "AxisBounds"=w528, "ticsAndGrids"=w531, "Axis"=w532, "ShowNumbers?"=w537, "ShowLabel?"=w536, "Axis Label"=w524, "DataSpan"=w526) -> ("String out"=w512:string)  [unwired: 6 in, 1 out]
              n181 = Concatenate Strings(w512, w544) -> (w545:string)
            }
          }
          n182 = case shown="\"Polar\"" w433 {
            tunnel: w436 -> [w465 w470]
            tunnel: [w465 w469] -> w434
            tunnel: w432 -> [_ w467]
            frame "XY", Default {
            }
            frame "Polar" {
              n183 = local read "AngleMode"() -> (w468:string)
              n184 = call "MakeThetaLabels.vi"("AngleMode"=w468, "ticsAndGrids"=w467) -> ("Theta Label Command String"=w466:string)
              n185 = Concatenate Strings(w470, w466) -> (w469:string)
            }
          }
        }
        n186 = Concatenate Strings(w412, w413, "\nunset multiplot\n") -> (w418:string)
      }
      frame "Write gnuplot file" {
        w563 = FALSE  # append to file? (new file:F)
        w564 = FALSE  # advisory dialog? (display:T)
        n187 = Strip Path(path=w560) -> (stripped path=w557:path)  [unwired: 1 out]
        n188 = Build Path(base path=w557, name or relative path="gnuplot_script.txt") -> (appended path=w565:path)
        n189 = call "Write_Characters_To_File.vi"("file path (dialog if empty)"=w565, "advisory dialog? (display:T)"=w564, "character string"=w556, "append to file? (new file:F)"=w563) -> ()  [unwired: 1 in, 4 out]
      }
      frame "Execute shell script" {
        n190 = call "Run_Gnuplot_Script.vi"("logfileName"=w567, "workingDirectory"=w568) -> ()  [unwired: 1 in]
      }
      frame "Has pdf been generated?" {
        n191 = Seconds To Date/Time() -> (date time rec=w575:T18)  [unwired: 2 in]
        n192 = Strip Path(path=w597) -> (stripped path=w593:path, name=w596:string)
        n193 = Unbundle By Name(w575) -> ("year"=w576:i32, "month"=w577:i32, "day of month"=w578:i32)
        n194 = Strip Path(path=w593) -> (stripped path=w589:path)  [unwired: 1 out]
        n195 = Strip Path(path=w589) -> (stripped path=w585:path, name=w588:string)
        n196 = Concatenate Strings(w596, ".pdf" ("string")) -> (w594:string)
        n197 = Format Into String(format string="%d_M%02d_D%02d", w576, w577, w578) -> (resulting string=w574:string)  [unwired: 2 in, 1 out]
        n198 = Concatenate Strings(w588, ".pdf" ("string")) -> (w582:string)
        n199 = Build Path(base path=w593, name or relative path=w594) -> (appended path=w590:path)
        n200 = Build Path(base path=w585, name or relative path="Plot_pdfs") -> (appended path=w583:path)
        n201 = Current VI's Path() -> (path=w586:path)
        n202 = Build Path(base path=w583, name or relative path=w574) -> (appended path=w581:path)
        n203 = Build Path(base path=w581, name or relative path=w582) -> (appended path=w580:path)
        n204 = call "Running_as_top_level.vi"("Vi path name"=w586) -> ("Top Level"=w591:bool)  [unwired: 1 out]
        n205 = case shown="False" w591 {
          tunnel: w580 -> [w611 w613]
          tunnel: [w609 w612] -> w592
          frame False {
            n206 = call "Find_Unique_Filename.vi"("Path In"=w611) -> ("Unique Path Out"=w610:path)  [unwired: 2 in]
            n207 = call "Create_directory_path.vi"("Path name"=w610) -> ("Path name Out"=w609:path)  [unwired: 1 in, 1 out]
          }
          frame True {
            n208 = Delete(path (use dialog)=w613) -> (deleted path=w612:path)  [unwired: 4 in, 2 out]
          }
        }
        n209 = Select(t="Open Standard output file" ("f"), s="OpenLogfile?", f="End") -> (s? t:f=w598:string)
        n210 = Copy(10:w592, 11:w590) -> ()  [unwired: 3 in, 3 out]
        n211 = Select(t="Show Re-Run Gnuplot?", s="Show Script Editor?", f=w598) -> (s? t:f=w602:string)
      }
      frame "Show Re-Run Gnuplot?" {
        n212 = Strip Path(path=w615) -> (stripped path=w614:path)  [unwired: 1 out]
        n213 = call "Re_run_Gnuplot.vi"("Plot folder (dialog if empty)"=w614) -> ()  [unwired: 1 in, 3 out]
      }
      frame "Open Standard output file" {
        n214 = Strip Path(path=w625) -> (stripped path=w622:path)  [unwired: 1 out]
        n215 = Format Into String(format string="open \"%s\"", w623) -> (resulting string=w621:string)  [unwired: 2 in, 1 out]
        n216 = call <vilib>:"System Exec.vi"("working directory"=w622, "command line"=w621) -> ()  [unwired: 4 in, 6 out]
      }
      frame "End" {
      }
    }
    "gnuplotScript" <- w19
  }
  "AuditTrail" <- w5
  "Saved Automatically?" <- FALSE
